vi "Grid_multiGrid_v8.vi"() -> ()   [LabVIEW 2014]
uses:
  <userlib>/Nanonis Prog Interface V5/Nanonis Prog Interface.lvlib
panel:
  out "size(s) 5":i32
  out "size(s) 4":i32
  out "size(s) 3":i32=11
  out "size(s) 2":i32=12
  out "size(s)":i32=15
  out "data\n\n 5":T1(array[cluster])=[{"Amplitude (mod. signal unit)"=0.0, "Lockin on/off status"=FALSE, "Backward sweep"=TRUE, "Number of points"=215, "Channels"=["Current (A)", "LI Demod 1 X (A)", "LI Demod 1 Y (A)", "LI Demod 2 X (A)", "LI Demod 2 Y (A)"], "Parameters"=["X (m)", "Y (m)", "Z (m)", "Z offset (m)", "Settling time (s)", "Integration time (s)", "Z-Ctrl hold", "Final Z (m)"], "Fixed parameters"=["Sweep Start", "Sweep End"], "Multiple sweeps configuration"={"Number of Sweeps"=1, "Save all"=FALSE}, "Initialization"={"Z averaging time (s)"=0.001, "Initial settling time (s)"=0.0002}, "Sweep Timing"={"Max. slew rate (V/s)"=inf, "Settling time (s)"=0.001, "Integration time (s)"=0.001}, "End of Sweep"={"End settling time (s)"=5e-05, "Z control time (s)"=0.0002}, "Initial Z-Offset (m)"=0.0, "Sweep Distance (m)"=0.0, "Channels 2"=[], "Name"="", "Reset Z"=FALSE, "Record final Z"=FALSE, "Auto Retract Status"=FALSE, "Threshold"=0.0, "Auto Retract Signal Index"=0, "Auto Retract Condition"=FALSE}, {"Amplitude (mod. signal unit)"=0.0, "Lockin on/off status"=FALSE, "Backward sweep"=FALSE, "Number of points"=0, "Channels"=[], "Parameters"=[], "Fixed parameters"=[], "Multiple sweeps configuration"={"Number of Sweeps"=0, "Save all"=FALSE}, "Initialization"={"Z averaging time (s)"=0.0, "Initial settling time (s)"=0.0}, "Sweep Timing"={"Max. slew rate (V/s)"=0.0, "Settling time (s)"=0.0, "Integration time (s)"=0.0}, "End of Sweep"={"End settling time (s)"=0.0, "Z control time (s)"=0.0}, "Initial Z-Offset (m)"=0.0, "Sweep Distance (m)"=0.0, "Channels 2"=[], "Name"="", "Reset Z"=FALSE, "Record final Z"=FALSE, "Auto Retract Status"=FALSE, "Threshold"=0.0, "Auto Retract Signal Index"=0, "Auto Retract Condition"=FALSE}, {"Amplitude (mod. signal unit)"=0.0, "Lockin on/off status"=FALSE, "Backward sweep"=FALSE, "Number of points"=0, "Channels"=[], "Parameters"=[], "Fixed parameters"=[], "Multiple sweeps configuration"={"Number of Sweeps"=0, "Save all"=FALSE}, "Initialization"={"Z averaging time (s)"=0.0, "Initial settling time (s)"=0.0}, "Sweep Timing"={"Max. slew rate (V/s)"=0.0, "Settling time (s)"=0.0, "Integration time (s)"=0.0}, "End of Sweep"={"End settling time (s)"=0.0, "Z control time (s)"=0.0}, "Initial Z-Offset (m)"=0.0, "Sweep Distance (m)"=0.0, "Channels 2"=[], "Name"="", "Reset Z"=FALSE, "Record final Z"=FALSE, "Auto Retract Status"=FALSE, "Threshold"=0.0, "Auto Retract Signal Index"=0, "Auto Retract Condition"=FALSE}, {"Amplitude (mod. signal unit)"=0.0, "Lockin on/off status"=FALSE, "Backward sweep"=FALSE, "Number of points"=0, "Channels"=[], "Parameters"=[], "Fixed parameters"=[], "Multiple sweeps configuration"={"Number of Sweeps"=0, "Save all"=FALSE}, "Initialization"={"Z averaging time (s)"=0.0, "Initial settling time (s)"=0.0}, "Sweep Timing"={"Max. slew rate (V/s)"=0.0, "Settling time (s)"=0.0, "Integration time (s)"=0.0}, "End of Sweep"={"End settling time (s)"=0.0, "Z control time (s)"=0.0}, "Initial Z-Offset (m)"=0.0, "Sweep Distance (m)"=0.0, "Channels 2"=[], "Name"="", "Reset Z"=FALSE, "Record final Z"=FALSE, "Auto Retract Status"=FALSE, "Threshold"=0.0, "Auto Retract Signal Index"=0, "Auto Retract Condition"=FALSE}, {"Amplitude (mod. signal unit)"=0.0, "Lockin on/off status"=FALSE, "Backward sweep"=FALSE, "Number of points"=0, "Channels"=[], "Parameters"=[], "Fixed parameters"=[], "Multiple sweeps configuration"={"Number of Sweeps"=0, "Save all"=FALSE}, "Initialization"={"Z averaging time (s)"=0.0, "Initial settling time (s)"=0.0}, "Sweep Timing"={"Max. slew rate (V/s)"=0.0, "Settling time (s)"=0.0, "Integration time (s)"=0.0}, "End of Sweep"={"End settling time (s)"=0.0, "Z control time (s)"=0.0}, "Initial Z-Offset (m)"=0.0, "Sweep Distance (m)"=0.0, "Channels 2"=[], "Name"="", "Reset Z"=FALSE, "Record final Z"=FALSE, "Auto Retract Status"=FALSE, "Threshold"=0.0, "Auto Retract Signal Index"=0, "Auto Retract Condition"=FALSE}, {"Amplitude (mod. signal unit)"=0.0, "Lockin on/off status"=FALSE, "Backward sweep"=FALSE, "Number of points"=0, "Channels"=[], "Parameters"=[], "Fixed parameters"=[], "Multiple sweeps configuration"={"Number of Sweeps"=0, "Save all"=FALSE}, "Initialization"={"Z averaging time (s)"=0.0, "Initial settling time (s)"=0.0}, "Sweep Timing"={"Max. slew rate (V/s)"=0.0, "Settling time (s)"=0.0, "Integration time (s)"=0.0}, "End of Sweep"={"End settling time (s)"=0.0, "Z control time (s)"=0.0}, "Initial Z-Offset (m)"=0.0, "Sweep Distance (m)"=0.0, "Channels 2"=[], "Name"="", "Reset Z"=FALSE, "Record final Z"=FALSE, "Auto Retract Status"=FALSE, "Threshold"=0.0, "Auto Retract Signal Index"=0, "Auto Retract Condition"=FALSE}, {"Amplitude (mod. signal unit)"=0.0, "Lockin on/off status"=FALSE, "Backward sweep"=FALSE, "Number of points"=0, "Channels"=[], "Parameters"=[], "Fixed parameters"=[], "Multiple sweeps configuration"={"Number of Sweeps"=0, "Save all"=FALSE}, "Initialization"={"Z averaging time (s)"=0.0, "Initial settling time (s)"=0.0}, "Sweep Timing"={"Max. slew rate (V/s)"=0.0, "Settling time (s)"=0.0, "Integration time (s)"=0.0}, "End of Sweep"={"End settling time (s)"=0.0, "Z control time (s)"=0.0}, "Initial Z-Offset (m)"=0.0, "Sweep Distance (m)"=0.0, "Channels 2"=[], "Name"="", "Reset Z"=FALSE, "Record final Z"=FALSE, "Auto Retract Status"=FALSE, "Threshold"=0.0, "Auto Retract Signal Index"=0, "Auto Retract Condition"=FALSE}, {"Amplitude (mod. signal unit)"=0.0, "Lockin on/off status"=FALSE, "Backward sweep"=FALSE, "Number of points"=0, "Channels"=[], "Parameters"=[], "Fixed parameters"=[], "Multiple sweeps configuration"={"Number of Sweeps"=0, "Save all"=FALSE}, "Initialization"={"Z averaging time (s)"=0.0, "Initial settling time (s)"=0.0}, "Sweep Timing"={"Max. slew rate (V/s)"=0.0, "Settling time (s)"=0.0, "Integration time (s)"=0.0}, "End of Sweep"={"End settling time (s)"=0.0, "Z control time (s)"=0.0}, "Initial Z-Offset (m)"=0.0, "Sweep Distance (m)"=0.0, "Channels 2"=[], "Name"="", "Reset Z"=FALSE, "Record final Z"=FALSE, "Auto Retract Status"=FALSE, "Threshold"=0.0, "Auto Retract Signal Index"=0, "Auto Retract Condition"=FALSE}, {"Amplitude (mod. signal unit)"=0.0, "Lockin on/off status"=FALSE, "Backward sweep"=FALSE, "Number of points"=0, "Channels"=[], "Parameters"=[], "Fixed parameters"=[], "Multiple sweeps configuration"={"Number of Sweeps"=0, "Save all"=FALSE}, "Initialization"={"Z averaging time (s)"=0.0, "Initial settling time (s)"=0.0}, "Sweep Timing"={"Max. slew rate (V/s)"=0.0, "Settling time (s)"=0.0, "Integration time (s)"=0.0}, "End of Sweep"={"End settling time (s)"=0.0, "Z control time (s)"=0.0}, "Initial Z-Offset (m)"=0.0, "Sweep Distance (m)"=0.0, "Channels 2"=[], "Name"="", "Reset Z"=FALSE, "Record final Z"=FALSE, "Auto Retract Status"=FALSE, "Threshold"=0.0, "Auto Retract Signal Index"=0, "Auto Retract Condition"=FALSE}, {"Amplitude (mod. signal unit)"=0.0, "Lockin on/off status"=FALSE, "Backward sweep"=FALSE, "Number of points"=0, "Channels"=[], "Parameters"=[], "Fixed parameters"=[], "Multiple sweeps configuration"={"Number of Sweeps"=0, "Save all"=FALSE}, "Initialization"={"Z averaging time (s)"=0.0, "Initial settling time (s)"=0.0}, "Sweep Timing"={"Max. slew rate (V/s)"=0.0, "Settling time (s)"=0.0, "Integration time (s)"=0.0}, "End of Sweep"={"End settling time (s)"=0.0, "Z control time (s)"=0.0}, "Initial Z-Offset (m)"=0.0, "Sweep Distance (m)"=0.0, "Channels 2"=[], "Name"="", "Reset Z"=FALSE, "Record final Z"=FALSE, "Auto Retract Status"=FALSE, "Threshold"=0.0, "Auto Retract Signal Index"=0, "Auto Retract Condition"=FALSE}, {"Amplitude (mod. signal unit)"=0.0, "Lockin on/off status"=FALSE, "Backward sweep"=FALSE, "Number of points"=0, "Channels"=[], "Parameters"=[], "Fixed parameters"=[], "Multiple sweeps configuration"={"Number of Sweeps"=0, "Save all"=FALSE}, "Initialization"={"Z averaging time (s)"=0.0, "Initial settling time (s)"=0.0}, "Sweep Timing"={"Max. slew rate (V/s)"=0.0, "Settling time (s)"=0.0, "Integration time (s)"=0.0}, "End of Sweep"={"End settling time (s)"=0.0, "Z control time (s)"=0.0}, "Initial Z-Offset (m)"=0.0, "Sweep Distance (m)"=0.0, "Channels 2"=[], "Name"="", "Reset Z"=FALSE, "Record final Z"=FALSE, "Auto Retract Status"=FALSE, "Threshold"=0.0, "Auto Retract Signal Index"=0, "Auto Retract Condition"=FALSE}, {"Amplitude (mod. signal unit)"=0.0, "Lockin on/off status"=FALSE, "Backward sweep"=FALSE, "Number of points"=0, "Channels"=[], "Parameters"=[], "Fixed parameters"=[], "Multiple sweeps configuration"={"Number of Sweeps"=0, "Save all"=FALSE}, "Initialization"={"Z averaging time (s)"=0.0, "Initial settling time (s)"=0.0}, "Sweep Timing"={"Max. slew rate (V/s)"=0.0, "Settling time (s)"=0.0, "Integration time (s)"=0.0}, "End of Sweep"={"End settling time (s)"=0.0, "Z control time (s)"=0.0}, "Initial Z-Offset (m)"=0.0, "Sweep Distance (m)"=0.0, "Channels 2"=[], "Name"="", "Reset Z"=FALSE, "Record final Z"=FALSE, "Auto Retract Status"=FALSE, "Threshold"=0.0, "Auto Retract Signal Index"=0, "Auto Retract Condition"=FALSE}, {"Amplitude (mod. signal unit)"=0.0, "Lockin on/off status"=FALSE, "Backward sweep"=FALSE, "Number of points"=0, "Channels"=[], "Parameters"=[], "Fixed parameters"=[], "Multiple sweeps configuration"={"Number of Sweeps"=0, "Save all"=FALSE}, "Initialization"={"Z averaging time (s)"=0.0, "Initial settling time (s)"=0.0}, "Sweep Timing"={"Max. slew rate (V/s)"=0.0, "Settling time (s)"=0.0, "Integration time (s)"=0.0}, "End of Sweep"={"End settling time (s)"=0.0, "Z control time (s)"=0.0}, "Initial Z-Offset (m)"=0.0, "Sweep Distance (m)"=0.0, "Channels 2"=[], "Name"="", "Reset Z"=FALSE, "Record final Z"=FALSE, "Auto Retract Status"=FALSE, "Threshold"=0.0, "Auto Retract Signal Index"=0, "Auto Retract Condition"=FALSE}, {"Amplitude (mod. signal unit)"=0.0, "Lockin on/off status"=FALSE, "Backward sweep"=FALSE, "Number of points"=0, "Channels"=[], "Parameters"=[], "Fixed parameters"=[], "Multiple sweeps configuration"={"Number of Sweeps"=0, "Save all"=FALSE}, "Initialization"={"Z averaging time (s)"=0.0, "Initial settling time (s)"=0.0}, "Sweep Timing"={"Max. slew rate (V/s)"=0.0, "Settling time (s)"=0.0, "Integration time (s)"=0.0}, "End of Sweep"={"End settling time (s)"=0.0, "Z control time (s)"=0.0}, "Initial Z-Offset (m)"=0.0, "Sweep Distance (m)"=0.0, "Channels 2"=[], "Name"="", "Reset Z"=FALSE, "Record final Z"=FALSE, "Auto Retract Status"=FALSE, "Threshold"=0.0, "Auto Retract Signal Index"=0, "Auto Retract Condition"=FALSE}, {"Amplitude (mod. signal unit)"=0.0, "Lockin on/off status"=FALSE, "Backward sweep"=FALSE, "Number of points"=0, "Channels"=[], "Parameters"=[], "Fixed parameters"=[], "Multiple sweeps configuration"={"Number of Sweeps"=0, "Save all"=FALSE}, "Initialization"={"Z averaging time (s)"=0.0, "Initial settling time (s)"=0.0}, "Sweep Timing"={"Max. slew rate (V/s)"=0.0, "Settling time (s)"=0.0, "Integration time (s)"=0.0}, "End of Sweep"={"End settling time (s)"=0.0, "Z control time (s)"=0.0}, "Initial Z-Offset (m)"=0.0, "Sweep Distance (m)"=0.0, "Channels 2"=[], "Name"="", "Reset Z"=FALSE, "Record final Z"=FALSE, "Auto Retract Status"=FALSE, "Threshold"=0.0, "Auto Retract Signal Index"=0, "Auto Retract Condition"=FALSE}, {"Amplitude (mod. signal unit)"=0.0, "Lockin on/off status"=FALSE, "Backward sweep"=FALSE, "Number of points"=0, "Channels"=[], "Parameters"=[], "Fixed parameters"=[], "Multiple sweeps configuration"={"Number of Sweeps"=0, "Save all"=FALSE}, "Initialization"={"Z averaging time (s)"=0.0, "Initial settling time (s)"=0.0}, "Sweep Timing"={"Max. slew rate (V/s)"=0.0, "Settling time (s)"=0.0, "Integration time (s)"=0.0}, "End of Sweep"={"End settling time (s)"=0.0, "Z control time (s)"=0.0}, "Initial Z-Offset (m)"=0.0, "Sweep Distance (m)"=0.0, "Channels 2"=[], "Name"="", "Reset Z"=FALSE, "Record final Z"=FALSE, "Auto Retract Status"=FALSE, "Threshold"=0.0, "Auto Retract Signal Index"=0, "Auto Retract Condition"=FALSE}, {"Amplitude (mod. signal unit)"=0.0, "Lockin on/off status"=FALSE, "Backward sweep"=FALSE, "Number of points"=0, "Channels"=[], "Parameters"=[], "Fixed parameters"=[], "Multiple sweeps configuration"={"Number of Sweeps"=0, "Save all"=FALSE}, "Initialization"={"Z averaging time (s)"=0.0, "Initial settling time (s)"=0.0}, "Sweep Timing"={"Max. slew rate (V/s)"=0.0, "Settling time (s)"=0.0, "Integration time (s)"=0.0}, "End of Sweep"={"End settling time (s)"=0.0, "Z control time (s)"=0.0}, "Initial Z-Offset (m)"=0.0, "Sweep Distance (m)"=0.0, "Channels 2"=[], "Name"="", "Reset Z"=FALSE, "Record final Z"=FALSE, "Auto Retract Status"=FALSE, "Threshold"=0.0, "Auto Retract Signal Index"=0, "Auto Retract Condition"=FALSE}, {"Amplitude (mod. signal unit)"=0.0, "Lockin on/off status"=FALSE, "Backward sweep"=FALSE, "Number of points"=0, "Channels"=[], "Parameters"=[], "Fixed parameters"=[], "Multiple sweeps configuration"={"Number of Sweeps"=0, "Save all"=FALSE}, "Initialization"={"Z averaging time (s)"=0.0, "Initial settling time (s)"=0.0}, "Sweep Timing"={"Max. slew rate (V/s)"=0.0, "Settling time (s)"=0.0, "Integration time (s)"=0.0}, "End of Sweep"={"End settling time (s)"=0.0, "Z control time (s)"=0.0}, "Initial Z-Offset (m)"=0.0, "Sweep Distance (m)"=0.0, "Channels 2"=[], "Name"="", "Reset Z"=FALSE, "Record final Z"=FALSE, "Auto Retract Status"=FALSE, "Threshold"=0.0, "Auto Retract Signal Index"=0, "Auto Retract Condition"=FALSE}]
  out "data\n\n 2":T2(array[cluster])=[{"Amplitude (mod. signal unit)"=0.0, "Lockin on/off status"=FALSE, "Advanced options"={"Z-Controller Hold"=TRUE, "Record final Z"=FALSE, "Reset Bias"=TRUE}, "Backward sweep"=TRUE, "Number of points"=215, "Channels"=["Current (A)", "LI Demod 1 X (A)", "LI Demod 1 Y (A)", "LI Demod 2 X (A)", "LI Demod 2 Y (A)"], "Parameters"=["X (m)", "Y (m)", "Z (m)", "Z offset (m)", "Settling time (s)", "Integration time (s)", "Z-Ctrl hold", "Final Z (m)"], "Fixed parameters"=["Sweep Start", "Sweep End"], "Multiple sweeps configuration"={"Number of Sweeps"=1, "Save all"=FALSE}, "Initialization"={"Z averaging time (s)"=0.001, "Z offset (m)"=0.0, "Initial settling time (s)"=0.0002}, "Sweep Timing"={"Max. slew rate (V/s)"=inf, "Settling time (s)"=0.001, "Integration time (s)"=0.001}, "End of Sweep"={"End settling time (s)"=5e-05, "Z control time (s)"=0.0002}, "Start value (V)"=-0.02, "End value (V)"=-3.0, "Channels 2"=[0, 20, 21, 22, 23], "Name"="numerical_DCA_-20mV->-3V"}, {"Amplitude (mod. signal unit)"=0.0, "Lockin on/off status"=FALSE, "Advanced options"={"Z-Controller Hold"=TRUE, "Record final Z"=FALSE, "Reset Bias"=TRUE}, "Backward sweep"=TRUE, "Number of points"=215, "Channels"=["Current (A)", "LI Demod 1 X (A)", "LI Demod 1 Y (A)", "LI Demod 2 X (A)", "LI Demod 2 Y (A)"], "Parameters"=["X (m)", "Y (m)", "Z (m)", "Z offset (m)", "Settling time (s)", "Integration time (s)", "Z-Ctrl hold", "Final Z (m)"], "Fixed parameters"=["Sweep Start", "Sweep End"], "Multiple sweeps configuration"={"Number of Sweeps"=1, "Save all"=FALSE}, "Initialization"={"Z averaging time (s)"=0.001, "Z offset (m)"=0.0, "Initial settling time (s)"=0.0002}, "Sweep Timing"={"Max. slew rate (V/s)"=inf, "Settling time (s)"=0.001, "Integration time (s)"=0.001}, "End of Sweep"={"End settling time (s)"=5e-05, "Z control time (s)"=0.0002}, "Start value (V)"=-0.02, "End value (V)"=0.7, "Channels 2"=[0, 20, 21, 22, 23], "Name"="numerical_DCA_-20mV->0.7V"}, {"Amplitude (mod. signal unit)"=0.0, "Lockin on/off status"=FALSE, "Advanced options"={"Z-Controller Hold"=TRUE, "Record final Z"=FALSE, "Reset Bias"=TRUE}, "Backward sweep"=TRUE, "Number of points"=215, "Channels"=["Current (A)", "LI Demod 1 X (A)", "LI Demod 1 Y (A)", "LI Demod 2 X (A)", "LI Demod 2 Y (A)"], "Parameters"=["X (m)", "Y (m)", "Z (m)", "Z offset (m)", "Settling time (s)", "Integration time (s)", "Z-Ctrl hold", "Final Z (m)"], "Fixed parameters"=["Sweep Start", "Sweep End"], "Multiple sweeps configuration"={"Number of Sweeps"=30, "Save all"=FALSE}, "Initialization"={"Z averaging time (s)"=0.001, "Z offset (m)"=0.0, "Initial settling time (s)"=0.0002}, "Sweep Timing"={"Max. slew rate (V/s)"=inf, "Settling time (s)"=0.001, "Integration time (s)"=0.001}, "End of Sweep"={"End settling time (s)"=5e-05, "Z control time (s)"=0.0002}, "Start value (V)"=-0.02, "End value (V)"=0.7, "Channels 2"=[0, 20, 21, 22, 23], "Name"="numerical_DCA_-20mV->-0.7V_30sweeps"}, {"Amplitude (mod. signal unit)"=0.0, "Lockin on/off status"=FALSE, "Advanced options"={"Z-Controller Hold"=TRUE, "Record final Z"=FALSE, "Reset Bias"=TRUE}, "Backward sweep"=TRUE, "Number of points"=215, "Channels"=["Current (A)", "LI Demod 1 X (A)", "LI Demod 1 Y (A)", "LI Demod 2 X (A)", "LI Demod 2 Y (A)"], "Parameters"=["X (m)", "Y (m)", "Z (m)", "Z offset (m)", "Settling time (s)", "Integration time (s)", "Z-Ctrl hold", "Final Z (m)"], "Fixed parameters"=["Sweep Start", "Sweep End"], "Multiple sweeps configuration"={"Number of Sweeps"=50, "Save all"=FALSE}, "Initialization"={"Z averaging time (s)"=0.001, "Z offset (m)"=0.0, "Initial settling time (s)"=0.0002}, "Sweep Timing"={"Max. slew rate (V/s)"=inf, "Settling time (s)"=0.001, "Integration time (s)"=0.001}, "End of Sweep"={"End settling time (s)"=5e-05, "Z control time (s)"=0.0002}, "Start value (V)"=-0.02, "End value (V)"=0.7, "Channels 2"=[0, 20, 21, 22, 23], "Name"="numerical_DCA_-20mV->-0.7V_50_sweeps"}, {"Amplitude (mod. signal unit)"=0.0, "Lockin on/off status"=FALSE, "Advanced options"={"Z-Controller Hold"=TRUE, "Record final Z"=FALSE, "Reset Bias"=TRUE}, "Backward sweep"=TRUE, "Number of points"=215, "Channels"=["Current (A)", "LI Demod 1 X (A)", "LI Demod 1 Y (A)", "LI Demod 2 X (A)", "LI Demod 2 Y (A)"], "Parameters"=["X (m)", "Y (m)", "Z (m)", "Z offset (m)", "Settling time (s)", "Integration time (s)", "Z-Ctrl hold", "Final Z (m)"], "Fixed parameters"=["Sweep Start", "Sweep End"], "Multiple sweeps configuration"={"Number of Sweeps"=70, "Save all"=FALSE}, "Initialization"={"Z averaging time (s)"=0.001, "Z offset (m)"=0.0, "Initial settling time (s)"=0.0002}, "Sweep Timing"={"Max. slew rate (V/s)"=inf, "Settling time (s)"=0.001, "Integration time (s)"=0.001}, "End of Sweep"={"End settling time (s)"=5e-05, "Z control time (s)"=0.0002}, "Start value (V)"=-0.02, "End value (V)"=-3.0, "Channels 2"=[0, 20, 21, 22, 23], "Name"="numerical_DCA_-20mV->-3V_70sweeps"}, {"Amplitude (mod. signal unit)"=0.0, "Lockin on/off status"=FALSE, "Advanced options"={"Z-Controller Hold"=TRUE, "Record final Z"=FALSE, "Reset Bias"=TRUE}, "Backward sweep"=TRUE, "Number of points"=215, "Channels"=["Current (A)", "LI Demod 1 X (A)", "LI Demod 1 Y (A)", "LI Demod 2 X (A)", "LI Demod 2 Y (A)"], "Parameters"=["X (m)", "Y (m)", "Z (m)", "Z offset (m)", "Settling time (s)", "Integration time (s)", "Z-Ctrl hold", "Final Z (m)"], "Fixed parameters"=["Sweep Start", "Sweep End"], "Multiple sweeps configuration"={"Number of Sweeps"=100, "Save all"=FALSE}, "Initialization"={"Z averaging time (s)"=0.001, "Z offset (m)"=0.0, "Initial settling time (s)"=0.0002}, "Sweep Timing"={"Max. slew rate (V/s)"=inf, "Settling time (s)"=0.001, "Integration time (s)"=0.001}, "End of Sweep"={"End settling time (s)"=5e-05, "Z control time (s)"=0.0002}, "Start value (V)"=-0.02, "End value (V)"=-3.0, "Channels 2"=[0, 20, 21, 22, 23], "Name"="numerical_DCA_-20mV->3V_100_sweeps"}, {"Amplitude (mod. signal unit)"=0.0, "Lockin on/off status"=FALSE, "Advanced options"={"Z-Controller Hold"=TRUE, "Record final Z"=FALSE, "Reset Bias"=TRUE}, "Backward sweep"=TRUE, "Number of points"=256, "Channels"=["Current (A)", "LI Demod 1 X (A)", "LI Demod 1 Y (A)", "LI Demod 2 X (A)", "LI Demod 2 Y (A)"], "Parameters"=["X (m)", "Y (m)", "Z (m)", "Z offset (m)", "Settling time (s)", "Integration time (s)", "Z-Ctrl hold", "Final Z (m)"], "Fixed parameters"=["Sweep Start", "Sweep End"], "Multiple sweeps configuration"={"Number of Sweeps"=100, "Save all"=FALSE}, "Initialization"={"Z averaging time (s)"=0.001, "Z offset (m)"=0.0, "Initial settling time (s)"=5e-05}, "Sweep Timing"={"Max. slew rate (V/s)"=inf, "Settling time (s)"=0.001, "Integration time (s)"=0.0005}, "End of Sweep"={"End settling time (s)"=5e-05, "Z control time (s)"=5e-05}, "Start value (V)"=-1.0, "End value (V)"=2.0, "Channels 2"=[0, 20, 21, 22, 23], "Name"="numerical_-1V->2V"}, {"Amplitude (mod. signal unit)"=0.0, "Lockin on/off status"=FALSE, "Advanced options"={"Z-Controller Hold"=TRUE, "Record final Z"=FALSE, "Reset Bias"=TRUE}, "Backward sweep"=TRUE, "Number of points"=256, "Channels"=["Current (A)", "LI Demod 1 X (A)", "LI Demod 1 Y (A)", "LI Demod 2 X (A)", "LI Demod 2 Y (A)"], "Parameters"=["X (m)", "Y (m)", "Z (m)", "Z offset (m)", "Settling time (s)", "Integration time (s)", "Z-Ctrl hold", "Final Z (m)"], "Fixed parameters"=["Sweep Start", "Sweep End"], "Multiple sweeps configuration"={"Number of Sweeps"=100, "Save all"=FALSE}, "Initialization"={"Z averaging time (s)"=0.001, "Z offset (m)"=0.0, "Initial settling time (s)"=5e-05}, "Sweep Timing"={"Max. slew rate (V/s)"=inf, "Settling time (s)"=0.001, "Integration time (s)"=0.0005}, "End of Sweep"={"End settling time (s)"=5e-05, "Z control time (s)"=5e-05}, "Start value (V)"=-0.02, "End value (V)"=0.02, "Channels 2"=[0, 20, 21, 22, 23], "Name"="numerical_-20mV->20mV"}, {"Amplitude (mod. signal unit)"=0.0, "Lockin on/off status"=FALSE, "Advanced options"={"Z-Controller Hold"=TRUE, "Record final Z"=FALSE, "Reset Bias"=TRUE}, "Backward sweep"=TRUE, "Number of points"=286, "Channels"=["Current (A)", "LI Demod 1 X (A)", "LI Demod 1 Y (A)", "LI Demod 2 X (A)", "LI Demod 2 Y (A)"], "Parameters"=["X (m)", "Y (m)", "Z (m)", "Z offset (m)", "Settling time (s)", "Integration time (s)", "Z-Ctrl hold", "Final Z (m)"], "Fixed parameters"=["Sweep Start", "Sweep End"], "Multiple sweeps configuration"={"Number of Sweeps"=50, "Save all"=FALSE}, "Initialization"={"Z averaging time (s)"=0.001, "Z offset (m)"=0.0, "Initial settling time (s)"=5e-05}, "Sweep Timing"={"Max. slew rate (V/s)"=inf, "Settling time (s)"=0.001, "Integration time (s)"=0.0005}, "End of Sweep"={"End settling time (s)"=5e-05, "Z control time (s)"=5e-05}, "Start value (V)"=-0.2, "End value (V)"=0.8, "Channels 2"=[0, 20, 21, 22, 23], "Name"="DCA_numerical_-0.2V->0.8V"}, {"Amplitude (mod. signal unit)"=0.0, "Lockin on/off status"=FALSE, "Advanced options"={"Z-Controller Hold"=TRUE, "Record final Z"=FALSE, "Reset Bias"=TRUE}, "Backward sweep"=TRUE, "Number of points"=421, "Channels"=["Current (A)", "LI Demod 1 X (A)", "LI Demod 1 Y (A)", "LI Demod 2 X (A)", "LI Demod 2 Y (A)"], "Parameters"=["X (m)", "Y (m)", "Z (m)", "Z offset (m)", "Settling time (s)", "Integration time (s)", "Z-Ctrl hold", "Final Z (m)"], "Fixed parameters"=["Sweep Start", "Sweep End"], "Multiple sweeps configuration"={"Number of Sweeps"=100, "Save all"=FALSE}, "Initialization"={"Z averaging time (s)"=0.001, "Z offset (m)"=0.0, "Initial settling time (s)"=5e-05}, "Sweep Timing"={"Max. slew rate (V/s)"=inf, "Settling time (s)"=0.001, "Integration time (s)"=0.0005}, "End of Sweep"={"End settling time (s)"=5e-05, "Z control time (s)"=5e-05}, "Start value (V)"=-2.0, "End value (V)"=2.2, "Channels 2"=[0, 20, 21, 22, 23], "Name"="numerical_-2V->2.2V"}, {"Amplitude (mod. signal unit)"=0.0, "Lockin on/off status"=FALSE, "Advanced options"={"Z-Controller Hold"=TRUE, "Record final Z"=FALSE, "Reset Bias"=TRUE}, "Backward sweep"=TRUE, "Number of points"=500, "Channels"=["Current (A)", "LI Demod 1 X (A)", "LI Demod 1 Y (A)", "LI Demod 2 X (A)", "LI Demod 2 Y (A)"], "Parameters"=["X (m)", "Y (m)", "Z (m)", "Z offset (m)", "Settling time (s)", "Integration time (s)", "Z-Ctrl hold", "Final Z (m)"], "Fixed parameters"=["Sweep Start", "Sweep End"], "Multiple sweeps configuration"={"Number of Sweeps"=20, "Save all"=FALSE}, "Initialization"={"Z averaging time (s)"=0.001, "Z offset (m)"=0.0, "Initial settling time (s)"=0.01}, "Sweep Timing"={"Max. slew rate (V/s)"=inf, "Settling time (s)"=0.001, "Integration time (s)"=0.001}, "End of Sweep"={"End settling time (s)"=0.1, "Z control time (s)"=0.001}, "Start value (V)"=-0.2, "End value (V)"=0.8, "Channels 2"=[0, 20, 21, 22, 23], "Name"="DCA_numerical2_-0.2V->0.8V"}, {"Amplitude (mod. signal unit)"=0.0015, "Lockin on/off status"=FALSE, "Advanced options"={"Z-Controller Hold"=TRUE, "Record final Z"=FALSE, "Reset Bias"=TRUE}, "Backward sweep"=TRUE, "Number of points"=80, "Channels"=["Current (A)", "LI Demod 1 X (A)", "LI Demod 1 Y (A)", "LI Demod 2 X (A)", "LI Demod 2 Y (A)"], "Parameters"=["X (m)", "Y (m)", "Z (m)", "Z offset (m)", "Settling time (s)", "Integration time (s)", "Z-Ctrl hold", "Final Z (m)"], "Fixed parameters"=["Sweep Start", "Sweep End"], "Multiple sweeps configuration"={"Number of Sweeps"=10, "Save all"=FALSE}, "Initialization"={"Z averaging time (s)"=0.001, "Z offset (m)"=0.0, "Initial settling time (s)"=0.0046}, "Sweep Timing"={"Max. slew rate (V/s)"=inf, "Settling time (s)"=0.0046, "Integration time (s)"=0.032}, "End of Sweep"={"End settling time (s)"=5e-05, "Z control time (s)"=5e-05}, "Start value (V)"=-0.02, "End value (V)"=0.02, "Channels 2"=[0, 20, 21, 22, 23], "Name"="lockin_-20mV->20mV"}, {"Amplitude (mod. signal unit)"=0.002, "Lockin on/off status"=FALSE, "Advanced options"={"Z-Controller Hold"=TRUE, "Record final Z"=FALSE, "Reset Bias"=TRUE}, "Backward sweep"=TRUE, "Number of points"=70, "Channels"=["Current (A)", "LI Demod 1 X (A)", "LI Demod 1 Y (A)", "LI Demod 2 X (A)", "LI Demod 2 Y (A)"], "Parameters"=["X (m)", "Y (m)", "Z (m)", "Z offset (m)", "Settling time (s)", "Integration time (s)", "Z-Ctrl hold", "Final Z (m)"], "Fixed parameters"=["Sweep Start", "Sweep End"], "Multiple sweeps configuration"={"Number of Sweeps"=10, "Save all"=FALSE}, "Initialization"={"Z averaging time (s)"=0.001, "Z offset (m)"=0.0, "Initial settling time (s)"=0.0046}, "Sweep Timing"={"Max. slew rate (V/s)"=inf, "Settling time (s)"=0.0046, "Integration time (s)"=0.032}, "End of Sweep"={"End settling time (s)"=5e-05, "Z control time (s)"=5e-05}, "Start value (V)"=-0.025, "End value (V)"=0.025, "Channels 2"=[0, 20, 21, 22, 23], "Name"="lockin_-25mV->25mV"}, {"Amplitude (mod. signal unit)"=0.002, "Lockin on/off status"=FALSE, "Advanced options"={"Z-Controller Hold"=TRUE, "Record final Z"=FALSE, "Reset Bias"=TRUE}, "Backward sweep"=TRUE, "Number of points"=70, "Channels"=["Current (A)", "LI Demod 1 X (A)", "LI Demod 1 Y (A)", "LI Demod 2 X (A)", "LI Demod 2 Y (A)"], "Parameters"=["X (m)", "Y (m)", "Z (m)", "Z offset (m)", "Settling time (s)", "Integration time (s)", "Z-Ctrl hold", "Final Z (m)"], "Fixed parameters"=["Sweep Start", "Sweep End"], "Multiple sweeps configuration"={"Number of Sweeps"=10, "Save all"=FALSE}, "Initialization"={"Z averaging time (s)"=0.001, "Z offset (m)"=0.0, "Initial settling time (s)"=0.0046}, "Sweep Timing"={"Max. slew rate (V/s)"=inf, "Settling time (s)"=0.0046, "Integration time (s)"=0.032}, "End of Sweep"={"End settling time (s)"=5e-05, "Z control time (s)"=5e-05}, "Start value (V)"=-0.025, "End value (V)"=0.025, "Channels 2"=[0, 20, 21, 22, 23], "Name"="test"}, {"Amplitude (mod. signal unit)"=0.0025, "Lockin on/off status"=FALSE, "Advanced options"={"Z-Controller Hold"=TRUE, "Record final Z"=FALSE, "Reset Bias"=TRUE}, "Backward sweep"=TRUE, "Number of points"=320, "Channels"=["Current (A)", "LI Demod 1 X (A)", "LI Demod 1 Y (A)", "LI Demod 2 X (A)", "LI Demod 2 Y (A)"], "Parameters"=["X (m)", "Y (m)", "Z (m)", "Z offset (m)", "Settling time (s)", "Integration time (s)", "Z-Ctrl hold", "Final Z (m)"], "Fixed parameters"=["Sweep Start", "Sweep End"], "Multiple sweeps configuration"={"Number of Sweeps"=1, "Save all"=FALSE}, "Initialization"={"Z averaging time (s)"=0.001, "Z offset (m)"=0.0, "Initial settling time (s)"=0.0046}, "Sweep Timing"={"Max. slew rate (V/s)"=inf, "Settling time (s)"=0.0046, "Integration time (s)"=0.0042}, "End of Sweep"={"End settling time (s)"=5e-05, "Z control time (s)"=5e-05}, "Start value (V)"=0.02, "End value (V)"=-0.02, "Channels 2"=[0, 20, 21, 22, 23], "Name"="lockin_highRes_20mV_-20mV"}, {"Amplitude (mod. signal unit)"=0.005, "Lockin on/off status"=FALSE, "Advanced options"={"Z-Controller Hold"=TRUE, "Record final Z"=FALSE, "Reset Bias"=TRUE}, "Backward sweep"=TRUE, "Number of points"=256, "Channels"=["Current (A)", "LI Demod 1 X (A)", "LI Demod 1 Y (A)", "LI Demod 2 X (A)", "LI Demod 2 Y (A)"], "Parameters"=["X (m)", "Y (m)", "Z (m)", "Z offset (m)", "Settling time (s)", "Integration time (s)", "Z-Ctrl hold", "Final Z (m)"], "Fixed parameters"=["Sweep Start", "Sweep End"], "Multiple sweeps configuration"={"Number of Sweeps"=2, "Save all"=FALSE}, "Initialization"={"Z averaging time (s)"=0.001, "Z offset (m)"=0.0, "Initial settling time (s)"=0.0033}, "Sweep Timing"={"Max. slew rate (V/s)"=inf, "Settling time (s)"=0.0033, "Integration time (s)"=0.0164}, "End of Sweep"={"End settling time (s)"=5e-05, "Z control time (s)"=5e-05}, "Start value (V)"=-1.0, "End value (V)"=2.0, "Channels 2"=[0, 20, 21, 22, 23], "Name"="lockin_slow"}, {"Amplitude (mod. signal unit)"=0.005, "Lockin on/off status"=FALSE, "Advanced options"={"Z-Controller Hold"=TRUE, "Record final Z"=FALSE, "Reset Bias"=TRUE}, "Backward sweep"=TRUE, "Number of points"=310, "Channels"=["Current (A)", "LI Demod 1 X (A)", "LI Demod 1 Y (A)", "LI Demod 2 X (A)", "LI Demod 2 Y (A)"], "Parameters"=["X (m)", "Y (m)", "Z (m)", "Z offset (m)", "Settling time (s)", "Integration time (s)", "Z-Ctrl hold", "Final Z (m)"], "Fixed parameters"=["Sweep Start", "Sweep End"], "Multiple sweeps configuration"={"Number of Sweeps"=2, "Save all"=FALSE}, "Initialization"={"Z averaging time (s)"=0.001, "Z offset (m)"=0.0, "Initial settling time (s)"=0.0031}, "Sweep Timing"={"Max. slew rate (V/s)"=inf, "Settling time (s)"=0.0031, "Integration time (s)"=0.0246}, "End of Sweep"={"End settling time (s)"=5e-05, "Z control time (s)"=5e-05}, "Start value (V)"=1.5, "End value (V)"=-0.05, "Channels 2"=[0, 20, 21, 22, 23], "Name"="Lock_in_DCA_1.5V->-50mV"}, {"Amplitude (mod. signal unit)"=0.005, "Lockin on/off status"=FALSE, "Advanced options"={"Z-Controller Hold"=TRUE, "Record final Z"=FALSE, "Reset Bias"=TRUE}, "Backward sweep"=TRUE, "Number of points"=401, "Channels"=["Current (A)", "Z (m)", "LI Demod 1 X (A)", "LI Demod 1 Y (A)", "LI Demod 2 X (A)", "LI Demod 2 Y (A)"], "Parameters"=["X (m)", "Y (m)", "Z (m)", "Z offset (m)", "Settling time (s)", "Integration time (s)", "Z-Ctrl hold", "Final Z (m)"], "Fixed parameters"=["Sweep Start", "Sweep End"], "Multiple sweeps configuration"={"Number of Sweeps"=1, "Save all"=FALSE}, "Initialization"={"Z averaging time (s)"=0.001, "Z offset (m)"=0.0, "Initial settling time (s)"=0.004}, "Sweep Timing"={"Max. slew rate (V/s)"=inf, "Settling time (s)"=0.02, "Integration time (s)"=0.015}, "End of Sweep"={"End settling time (s)"=5e-05, "Z control time (s)"=0.001}, "Start value (V)"=-1.0, "End value (V)"=1.0, "Channels 2"=[0, 14, 20, 21, 22, 23], "Name"="Long_MgPc_lockin_-1->1V"}, {"Amplitude (mod. signal unit)"=0.005, "Lockin on/off status"=FALSE, "Advanced options"={"Z-Controller Hold"=TRUE, "Record final Z"=FALSE, "Reset Bias"=TRUE}, "Backward sweep"=TRUE, "Number of points"=467, "Channels"=["Current (A)", "Z (m)", "LI Demod 1 X (A)", "LI Demod 1 Y (A)", "LI Demod 2 X (A)", "LI Demod 2 Y (A)"], "Parameters"=["X (m)", "Y (m)", "Z (m)", "Z offset (m)", "Settling time (s)", "Integration time (s)", "Z-Ctrl hold", "Final Z (m)"], "Fixed parameters"=["Sweep Start", "Sweep End"], "Multiple sweeps configuration"={"Number of Sweeps"=2, "Save all"=FALSE}, "Initialization"={"Z averaging time (s)"=0.001, "Z offset (m)"=0.0, "Initial settling time (s)"=0.004}, "Sweep Timing"={"Max. slew rate (V/s)"=inf, "Settling time (s)"=0.02, "Integration time (s)"=0.0246}, "End of Sweep"={"End settling time (s)"=5e-05, "Z control time (s)"=0.001}, "Start value (V)"=-2.0, "End value (V)"=1.5, "Channels 2"=[0, 14, 20, 21, 22, 23], "Name"="MgPc_long_lockin"}, {"Amplitude (mod. signal unit)"=0.008, "Lockin on/off status"=FALSE, "Advanced options"={"Z-Controller Hold"=TRUE, "Record final Z"=FALSE, "Reset Bias"=TRUE}, "Backward sweep"=TRUE, "Number of points"=256, "Channels"=["Current (A)", "LI Demod 1 X (A)", "LI Demod 1 Y (A)", "LI Demod 2 X (A)", "LI Demod 2 Y (A)"], "Parameters"=["X (m)", "Y (m)", "Z (m)", "Z offset (m)", "Settling time (s)", "Integration time (s)", "Z-Ctrl hold", "Final Z (m)"], "Fixed parameters"=["Sweep Start", "Sweep End"], "Multiple sweeps configuration"={"Number of Sweeps"=3, "Save all"=FALSE}, "Initialization"={"Z averaging time (s)"=0.001, "Z offset (m)"=0.0, "Initial settling time (s)"=0.0033}, "Sweep Timing"={"Max. slew rate (V/s)"=inf, "Settling time (s)"=0.0033, "Integration time (s)"=0.0082}, "End of Sweep"={"End settling time (s)"=5e-05, "Z control time (s)"=5e-05}, "Start value (V)"=-1.0, "End value (V)"=2.0, "Channels 2"=[0, 20, 21, 22, 23], "Name"="lockin_slow_-1_2"}, {"Amplitude (mod. signal unit)"=0.008, "Lockin on/off status"=FALSE, "Advanced options"={"Z-Controller Hold"=TRUE, "Record final Z"=FALSE, "Reset Bias"=TRUE}, "Backward sweep"=TRUE, "Number of points"=421, "Channels"=["Current (A)", "Z (m)", "LI Demod 1 X (A)", "LI Demod 1 Y (A)", "LI Demod 2 X (A)", "LI Demod 2 Y (A)"], "Parameters"=["X (m)", "Y (m)", "Z (m)", "Z offset (m)", "Settling time (s)", "Integration time (s)", "Z-Ctrl hold", "Final Z (m)"], "Fixed parameters"=["Sweep Start", "Sweep End"], "Multiple sweeps configuration"={"Number of Sweeps"=2, "Save all"=FALSE}, "Initialization"={"Z averaging time (s)"=0.001, "Z offset (m)"=0.0, "Initial settling time (s)"=5e-05}, "Sweep Timing"={"Max. slew rate (V/s)"=inf, "Settling time (s)"=0.0164, "Integration time (s)"=0.0164}, "End of Sweep"={"End settling time (s)"=5e-05, "Z control time (s)"=0.001}, "Start value (V)"=-2.0, "End value (V)"=2.2, "Channels 2"=[0, 14, 20, 21, 22, 23], "Name"="MgPc_long_lockin2"}, {"Amplitude (mod. signal unit)"=0.01, "Lockin on/off status"=FALSE, "Advanced options"={"Z-Controller Hold"=TRUE, "Record final Z"=FALSE, "Reset Bias"=TRUE}, "Backward sweep"=TRUE, "Number of points"=512, "Channels"=["Current (A)", "LI Demod 1 X (A)", "LI Demod 1 Y (A)", "LI Demod 2 X (A)", "LI Demod 2 Y (A)"], "Parameters"=["X (m)", "Y (m)", "Z (m)", "Z offset (m)", "Settling time (s)", "Integration time (s)", "Z-Ctrl hold", "Final Z (m)"], "Fixed parameters"=["Sweep Start", "Sweep End"], "Multiple sweeps configuration"={"Number of Sweeps"=1, "Save all"=FALSE}, "Initialization"={"Z averaging time (s)"=0.001, "Z offset (m)"=0.0, "Initial settling time (s)"=0.2}, "Sweep Timing"={"Max. slew rate (V/s)"=inf, "Settling time (s)"=0.0082, "Integration time (s)"=0.041}, "End of Sweep"={"End settling time (s)"=5e-05, "Z control time (s)"=5e-05}, "Start value (V)"=-3.0, "End value (V)"=2.0, "Channels 2"=[0, 20, 21, 22, 23], "Name"="Quick_Lockin"}]
  in  "Save As":string
  in  "Zspecparam.txt location":path=path "D:/Scripts/STSparam - Copy (2).txt"
  in  "Save As 2":string
  in  "STSparam.txt location":path=path "D:/Scripts/STSparam.txt"
  in  "Update STS/Zspec Param List":bool
  in  "START EXPERIMENT":bool
  in  "stop":bool
  in  "Duplicate Page 1":bool
  in  "No. of Exp":dbl=2.0 caption="No. of Experiments \n(If more than 5, edit VI)" step=1.0
  in  "Tab Control":T3(tab)=enum."Page 2"
  in  "Experiment 1":T4={"Drift Correction Settings"={"Drift Correction every"=4, "Drift correction Pixels"=128, "Channel index (0-23)"=0, "MaxImagesBack"=2, "Threshold"=2, "Increment"=1, "max applied Drift Correction"=40, "Correct Drift"=TRUE, "Correlate"=0, "Correct z drift"=FALSE, "zdrift \nDuration (s)"=0.0}, "Spectroscopy Setting"={"Imaging Current"=5e-11, "ref Current"=5e-12, "tip Speed (m/s)"=2e-09, "Imaging Bias"=-2.4, "ref Bias"=-0.02, "preSTS delay [ms]"=500, "STS z offset"=2e-10, "during Spec Bias (V)"=-0.02, "trigger1 < Hz"=0.0, "trigger 2 >Hz"=0.0, "autoStop"=FALSE, "Spectroscopy"=0, "PLL ON/OFF"=FALSE, "readjust setpoint every "=1, "z Reference"=TRUE, "Lock In"=FALSE}, "Misc"={"File name"="DCA_Zdependence_STS_Neg_Bias_Mol5_1_zOffset=200pm", "Email when finished"="Dhaneesh.Gopalakrishnan@monash.edu"}, "Grid Settings"={"type"=0, "type order"=0, "X pixel"=6, "Y pixel"=1, "Grid_Parms"={"center X (m)"=0.0, "center Y (m)"=0.0, "width (m)"=0.0, "height (m)"=0.0, "angle (deg)"=0.0}}, "STS Param List #1 "=4, "ZSpec Param List #1  "=0, "Repeat Experiment"={"Repeat"=TRUE, "Repeat Parameter"=2, "Values List #1"=14}} {"Repeat Experiment"."Repeat Parameter" items=["ref Current", "ref Bias", "STS z offset", "during Spec Bias (V)"]; "STS Param List #1" items=["numerical_DCA_-20mV->-3V", "numerical_DCA_-20mV->0.7V", "numerical_DCA_-20mV->-3V_3sweeps", "numerical_DCA_-20mV->-0.7V_30sweeps", "numerical_DCA_-20mV->-3V_50sweeps", "numerical_DCA_-20mV->-0.7V_50_sweeps", "numerical_DCA_-20mV->-3V_70sweeps", "numerical_DCA_-20mV->3V_100_sweeps", "numerical_DCA_-1V_>-3.2V_10sweeps", "numerical_DCA_-1V_>-3.2V_50sweeps", "numerical_DCA_-200m->800mV_50sweeps", "numerical_-1V->2V", "numerical_-20mV->20mV", "numerical_DCA_150mV->400mV", "DCA_numerical_-0.2V->0.8V", "V_star4_-20mV->-3V_3sweeps", "numerical_DCA_-20mV->-3V_10sweeps", "V_star2_-20mV->-3V_3sweeps", "V_star3_-20mV->-3.2V_3sweeps", "V_star5_-20mV->-3.5V_35sweeps", "V_star1_-20mV->-3.5V_70sweeps", "numerical_DCA_-20mV->-0.7V_50_sweepsV2", "numerical_DCA_0.12V_>0.6V_50sweeps", "numerical_-2V->2.2V", "DCA_numerical2_-0.2V->0.8V", "numerical_DCA_-200m->800mV_50sweepsV2", "lockin_-20mV->20mV", "lockin_-25mV->25mV", "test", "lockin_highRes_20mV_-20mV", "lockin_slow", "Lock_in_DCA_1.5V->-50mV", "Long_MgPc_lockin_-1->1V", "MgPc_long_lockin", "lockin_slow_-1_2", "MgPc_long_lockin2", "Quick_Lockin"]; "Grid Settings"."type order" items=["Grid", "Random", "Adam7"]; "Grid Settings"."type" items=["Line", "Grid", "Cloud"]; "Spectroscopy Setting"."Spectroscopy" items=["Bias", "zSpec"]; "Spectroscopy Setting"."trigger 2 >Hz" format="%#_6p"; "Spectroscopy Setting"."trigger1 < Hz" format="%#_6p"; "Spectroscopy Setting"."during Spec Bias (V)" format="%#_5p"; "Spectroscopy Setting"."STS z offset" format="%#_6p"; "Spectroscopy Setting"."ref Bias" format="%#_6p"; "Spectroscopy Setting"."Imaging Bias" format="%#_6p"; "Spectroscopy Setting"."tip Speed (m/s)" format="%.2p"; "Spectroscopy Setting"."ref Current" format="%#_6p"; "Spectroscopy Setting"."Imaging Current" format="%#_6p"; "Drift Correction Settings"."Correlate" items=["first Frame", "successive Frames"]; "Drift Correction Settings"."max applied Drift Correction" min=1 max=100 step=1 format="%.0p"; "Drift Correction Settings"."Threshold" min=1 step=1; "Drift Correction Settings"."Channel index (0-23)" items=["Current"=0, "Z (m)"=14]}
  in  "Experiment 2":T5={"Drift Correction Settings"={"Drift Correction every"=1, "Drift correction Pixels"=128, "Channel index (0-23)"=0, "MaxImagesBack"=2, "Threshold"=2, "Increment"=1, "max applied Drift Correction"=40, "Correct Drift"=TRUE, "Correlate"=0, "Correct z drift"=FALSE, "zdrift \nDuration (s)"=0.0}, "Spectroscopy Setting"={"Imaging Current"=5e-11, "ref Current"=5e-12, "tip Speed (m/s)"=2e-09, "Imaging Bias"=-2.4, "ref Bias"=-0.02, "preSTS delay [ms]"=500, "STS z offset"=0.0, "during Spec Bias (V)"=-0.02, "trigger1 < Hz"=0.0, "trigger 2 >Hz"=0.0, "autoStop"=FALSE, "Spectroscopy"=0, "PLL ON/OFF"=FALSE, "readjust setpoint every "=1, "z Reference"=TRUE, "Lock In"=FALSE}, "Misc"={"File name"="DCA_Zdependence_STS_Neg_Bias_Mol5_1", "Email when finished"="Dhaneesh.Gopalakrishnan@monash.edu"}, "Grid Settings"={"type"=0, "type order"=0, "X pixel"=6, "Y pixel"=1, "Grid_Parms"={"center X (m)"=0.0, "center Y (m)"=0.0, "width (m)"=0.0, "height (m)"=0.0, "angle (deg)"=0.0}}, "STS Param List #2 "=0, "ZSpec Param List  #2 "=0, "Repeat Experiment"={"Repeat"=TRUE, "Repeat Parameter"=2, "Values List #2"=7}} {"Repeat Experiment"."Repeat Parameter" items=["ref Current", "ref Bias", "STS z offset", "during Spec Bias (V)"]; "STS Param List #2" items=["numerical_DCA_-20mV->-3V", "numerical_DCA_-20mV->0.7V", "numerical_DCA_-20mV->-3V_3sweeps", "numerical_DCA_-20mV->-0.7V_30sweeps", "numerical_DCA_-20mV->-3V_50sweeps", "numerical_DCA_-20mV->-0.7V_50_sweeps", "numerical_DCA_-20mV->-3V_70sweeps", "numerical_DCA_-20mV->3V_100_sweeps", "numerical_DCA_-1V_>-3.2V_10sweeps", "numerical_DCA_-1V_>-3.2V_50sweeps", "numerical_DCA_-200m->800mV_50sweeps", "numerical_-1V->2V", "numerical_-20mV->20mV", "numerical_DCA_150mV->400mV", "DCA_numerical_-0.2V->0.8V", "V_star4_-20mV->-3V_3sweeps", "numerical_DCA_-20mV->-3V_10sweeps", "V_star2_-20mV->-3V_3sweeps", "V_star3_-20mV->-3.2V_3sweeps", "V_star5_-20mV->-3.5V_35sweeps", "V_star1_-20mV->-3.5V_70sweeps", "numerical_DCA_-20mV->-0.7V_50_sweepsV2", "numerical_DCA_0.12V_>0.6V_50sweeps", "numerical_-2V->2.2V", "DCA_numerical2_-0.2V->0.8V", "numerical_DCA_-200m->800mV_50sweepsV2", "lockin_-20mV->20mV", "lockin_-25mV->25mV", "test", "lockin_highRes_20mV_-20mV", "lockin_slow", "Lock_in_DCA_1.5V->-50mV", "Long_MgPc_lockin_-1->1V", "MgPc_long_lockin", "lockin_slow_-1_2", "MgPc_long_lockin2", "Quick_Lockin"]; "Grid Settings"."type order" items=["Grid", "Random", "Adam7"]; "Grid Settings"."type" items=["Line", "Grid", "Cloud"]; "Spectroscopy Setting"."Spectroscopy" items=["Bias", "zSpec"]; "Spectroscopy Setting"."trigger 2 >Hz" format="%#_6p"; "Spectroscopy Setting"."trigger1 < Hz" format="%#_6p"; "Spectroscopy Setting"."during Spec Bias (V)" format="%#_5p"; "Spectroscopy Setting"."STS z offset" format="%#_6p"; "Spectroscopy Setting"."ref Bias" format="%#_6p"; "Spectroscopy Setting"."Imaging Bias" format="%#_6p"; "Spectroscopy Setting"."tip Speed (m/s)" format="%.2p"; "Spectroscopy Setting"."ref Current" format="%#_6p"; "Spectroscopy Setting"."Imaging Current" format="%#_6p"; "Drift Correction Settings"."Correlate" items=["first Frame", "successive Frames"]; "Drift Correction Settings"."max applied Drift Correction" min=1 max=100 step=1 format="%.0p"; "Drift Correction Settings"."Threshold" min=1 step=1; "Drift Correction Settings"."Channel index (0-23)" items=["Current"=0, "Z (m)"=14]}
  in  "Experiment 3":T6={"Drift Correction Settings"={"Drift Correction every"=6, "Drift correction Pixels"=128, "Channel index (0-23)"=0, "MaxImagesBack"=2, "Threshold"=2, "Increment"=1, "max applied Drift Correction"=40, "Correct Drift"=TRUE, "Correlate"=0, "Correct z drift"=FALSE, "zdrift \nDuration (s)"=0.0}, "Spectroscopy Setting"={"Imaging Current"=5e-11, "ref Current"=5e-12, "tip Speed (m/s)"=2e-09, "Imaging Bias"=-2.4, "ref Bias"=-0.02, "preSTS delay [ms]"=500, "STS z offset"=4e-10, "during Spec Bias (V)"=-0.02, "trigger1 < Hz"=0.0, "trigger 2 >Hz"=0.0, "autoStop"=FALSE, "Spectroscopy"=0, "PLL ON/OFF"=FALSE, "readjust setpoint every "=1, "z Reference"=TRUE, "Lock In"=FALSE}, "Misc"={"File name"="DCA_Zdependence_STS_Neg_Bias_Mol5_1", "Email when finished"="Dhaneesh.Gopalakrishnan@monash.edu"}, "Grid Settings"={"type"=0, "type order"=0, "X pixel"=6, "Y pixel"=1, "Grid_Parms"={"center X (m)"=0.0, "center Y (m)"=0.0, "width (m)"=0.0, "height (m)"=0.0, "angle (deg)"=0.0}}, "STS Param List #3 "=4, "ZSpec Param List #3 "=0, "Repeat Experiment"={"Repeat"=TRUE, "Repeat Parameter"=2, "Values List #3"=7}} {"Repeat Experiment"."Repeat Parameter" items=["ref Current", "ref Bias", "STS z offset", "during Spec Bias (V)"]; "STS Param List #3" items=["numerical_DCA_-20mV->-3V", "numerical_DCA_-20mV->0.7V", "numerical_DCA_-20mV->-3V_3sweeps", "numerical_DCA_-20mV->-0.7V_30sweeps", "numerical_DCA_-20mV->-3V_50sweeps", "numerical_DCA_-20mV->-0.7V_50_sweeps", "numerical_DCA_-20mV->-3V_70sweeps", "numerical_DCA_-20mV->3V_100_sweeps", "numerical_DCA_-1V_>-3.2V_10sweeps", "numerical_DCA_-1V_>-3.2V_50sweeps", "numerical_DCA_-200m->800mV_50sweeps", "numerical_-1V->2V", "numerical_-20mV->20mV", "numerical_DCA_150mV->400mV", "DCA_numerical_-0.2V->0.8V", "V_star4_-20mV->-3V_3sweeps", "numerical_DCA_-20mV->-3V_10sweeps", "V_star2_-20mV->-3V_3sweeps", "V_star3_-20mV->-3.2V_3sweeps", "V_star5_-20mV->-3.5V_35sweeps", "V_star1_-20mV->-3.5V_70sweeps", "numerical_DCA_-20mV->-0.7V_50_sweepsV2", "numerical_DCA_0.12V_>0.6V_50sweeps", "numerical_-2V->2.2V", "DCA_numerical2_-0.2V->0.8V", "numerical_DCA_-200m->800mV_50sweepsV2", "lockin_-20mV->20mV", "lockin_-25mV->25mV", "test", "lockin_highRes_20mV_-20mV", "lockin_slow", "Lock_in_DCA_1.5V->-50mV", "Long_MgPc_lockin_-1->1V", "MgPc_long_lockin", "lockin_slow_-1_2", "MgPc_long_lockin2", "Quick_Lockin"]; "Grid Settings"."type order" items=["Grid", "Random", "Adam7"]; "Grid Settings"."type" items=["Line", "Grid", "Cloud"]; "Spectroscopy Setting"."Spectroscopy" items=["Bias", "zSpec"]; "Spectroscopy Setting"."trigger 2 >Hz" format="%#_6p"; "Spectroscopy Setting"."trigger1 < Hz" format="%#_6p"; "Spectroscopy Setting"."during Spec Bias (V)" format="%#_5p"; "Spectroscopy Setting"."STS z offset" format="%#_6p"; "Spectroscopy Setting"."ref Bias" format="%#_6p"; "Spectroscopy Setting"."Imaging Bias" format="%#_6p"; "Spectroscopy Setting"."tip Speed (m/s)" format="%.2p"; "Spectroscopy Setting"."ref Current" format="%#_6p"; "Spectroscopy Setting"."Imaging Current" format="%#_6p"; "Drift Correction Settings"."Correlate" items=["first Frame", "successive Frames"]; "Drift Correction Settings"."max applied Drift Correction" min=1 max=100 step=1 format="%.0p"; "Drift Correction Settings"."Threshold" min=1 step=1; "Drift Correction Settings"."Channel index (0-23)" items=["Current"=0, "Z (m)"=14]}
  in  "Experiment 4":T7={"Drift Correction Settings"={"Drift Correction every"=1, "Drift correction Pixels"=128, "Channel index (0-23)"=0, "MaxImagesBack"=2, "Threshold"=2, "Increment"=1, "max applied Drift Correction"=40, "Correct Drift"=TRUE, "Correlate"=0, "Correct z drift"=FALSE, "zdrift \nDuration (s)"=0.0}, "Spectroscopy Setting"={"Imaging Current"=5e-11, "ref Current"=5e-12, "tip Speed (m/s)"=1e-08, "Imaging Bias"=-2.4, "ref Bias"=-0.02, "preSTS delay [ms]"=500, "STS z offset"=0.0, "during Spec Bias (V)"=-0.02, "trigger1 < Hz"=0.0, "trigger 2 >Hz"=0.0, "autoStop"=FALSE, "Spectroscopy"=0, "PLL ON/OFF"=FALSE, "readjust setpoint every "=1, "z Reference"=TRUE, "Lock In"=FALSE}, "Misc"={"File name"="DCA_Zdependence_STS_Neg_Bias_Mol5_1", "Email when finished"="Dhaneesh.Gopalakrishnan@monash.edu"}, "Grid Settings"={"type"=0, "type order"=0, "X pixel"=6, "Y pixel"=1, "Grid_Parms"={"center X (m)"=0.0, "center Y (m)"=0.0, "width (m)"=0.0, "height (m)"=0.0, "angle (deg)"=0.0}}, "STS Param List #4 "=0, "ZSpec Param List  #4"=0, "Repeat Experiment"={"Repeat"=TRUE, "Repeat Parameter"=2, "Values List #4"=7}} {"Repeat Experiment"."Repeat Parameter" items=["ref Current", "ref Bias", "STS z offset", "during Spec Bias (V)"]; "STS Param List #4" items=["numerical_DCA_-20mV->-3V", "numerical_DCA_-20mV->0.7V", "numerical_DCA_-20mV->-3V_3sweeps", "numerical_DCA_-20mV->-0.7V_30sweeps", "numerical_DCA_-20mV->-3V_50sweeps", "numerical_DCA_-20mV->-0.7V_50_sweeps", "numerical_DCA_-20mV->-3V_70sweeps", "numerical_DCA_-20mV->3V_100_sweeps", "numerical_DCA_-1V_>-3.2V_10sweeps", "numerical_DCA_-1V_>-3.2V_50sweeps", "numerical_DCA_-200m->800mV_50sweeps", "numerical_-1V->2V", "numerical_-20mV->20mV", "numerical_DCA_150mV->400mV", "DCA_numerical_-0.2V->0.8V", "V_star4_-20mV->-3V_3sweeps", "numerical_DCA_-20mV->-3V_10sweeps", "V_star2_-20mV->-3V_3sweeps", "V_star3_-20mV->-3.2V_3sweeps", "V_star5_-20mV->-3.5V_35sweeps", "V_star1_-20mV->-3.5V_70sweeps", "numerical_DCA_-20mV->-0.7V_50_sweepsV2", "numerical_DCA_0.12V_>0.6V_50sweeps", "numerical_-2V->2.2V", "DCA_numerical2_-0.2V->0.8V", "numerical_DCA_-200m->800mV_50sweepsV2", "lockin_-20mV->20mV", "lockin_-25mV->25mV", "test", "lockin_highRes_20mV_-20mV", "lockin_slow", "Lock_in_DCA_1.5V->-50mV", "Long_MgPc_lockin_-1->1V", "MgPc_long_lockin", "lockin_slow_-1_2", "MgPc_long_lockin2", "Quick_Lockin"]; "Grid Settings"."type order" items=["Grid", "Random", "Adam7"]; "Grid Settings"."type" items=["Line", "Grid", "Cloud"]; "Spectroscopy Setting"."Spectroscopy" items=["Bias", "zSpec"]; "Spectroscopy Setting"."trigger 2 >Hz" format="%#_6p"; "Spectroscopy Setting"."trigger1 < Hz" format="%#_6p"; "Spectroscopy Setting"."during Spec Bias (V)" format="%#_5p"; "Spectroscopy Setting"."STS z offset" format="%#_6p"; "Spectroscopy Setting"."ref Bias" format="%#_6p"; "Spectroscopy Setting"."Imaging Bias" format="%#_6p"; "Spectroscopy Setting"."tip Speed (m/s)" format="%.2p"; "Spectroscopy Setting"."ref Current" format="%#_6p"; "Spectroscopy Setting"."Imaging Current" format="%#_6p"; "Drift Correction Settings"."Correlate" items=["first Frame", "successive Frames"]; "Drift Correction Settings"."max applied Drift Correction" min=1 max=100 step=1 format="%.0p"; "Drift Correction Settings"."Threshold" min=1 step=1; "Drift Correction Settings"."Channel index (0-23)" items=["Current"=0, "Z (m)"=14]}
  in  "Experiment 5":T8={"Drift Correction Settings"={"Drift Correction every"=1, "Drift correction Pixels"=256, "Channel index (0-23)"=0, "MaxImagesBack"=2, "Threshold"=2, "Increment"=1, "max applied Drift Correction"=40, "Correct Drift"=TRUE, "Correlate"=0, "Correct z drift"=FALSE, "zdrift \nDuration (s)"=0.0}, "Spectroscopy Setting"={"Imaging Current"=5e-11, "ref Current"=5e-12, "tip Speed (m/s)"=1e-08, "Imaging Bias"=-2.4, "ref Bias"=-0.02, "preSTS delay [ms]"=500, "STS z offset"=0.0, "during Spec Bias (V)"=-0.02, "trigger1 < Hz"=0.0, "trigger 2 >Hz"=0.0, "autoStop"=FALSE, "Spectroscopy"=0, "PLL ON/OFF"=FALSE, "readjust setpoint every "=1, "z Reference"=TRUE, "Lock In"=FALSE}, "Misc"={"File name"="DCA_Zdependence_STS_Pos_Bias_Mol9_46", "Email when finished"="Dhaneesh.Gopalakrishnan@monash.edu"}, "Grid Settings"={"type"=0, "type order"=0, "X pixel"=27, "Y pixel"=1, "Grid_Parms"={"center X (m)"=0.0, "center Y (m)"=0.0, "width (m)"=0.0, "height (m)"=0.0, "angle (deg)"=0.0}}, "STS Param List #5 "=0, "ZSpec Param List #5  "=0, "Repeat Experiment"={"Repeat"=TRUE, "Repeat Parameter"=2, "Values List #5"=7}} {"Repeat Experiment"."Repeat Parameter" items=["ref Current", "ref Bias", "STS z offset", "during Spec Bias (V)"]; "STS Param List #5" items=["numerical_DCA_-20mV->-3V", "numerical_DCA_-20mV->0.7V", "numerical_DCA_-20mV->-3V_3sweeps", "numerical_DCA_-20mV->-0.7V_30sweeps", "numerical_DCA_-20mV->-3V_50sweeps", "numerical_DCA_-20mV->-0.7V_50_sweeps", "numerical_DCA_-20mV->-3V_70sweeps", "numerical_DCA_-20mV->3V_100_sweeps", "numerical_DCA_-1V_>-3.2V_10sweeps", "numerical_DCA_-1V_>-3.2V_50sweeps", "numerical_DCA_-200m->800mV_50sweeps", "numerical_-1V->2V", "numerical_-20mV->20mV", "numerical_DCA_150mV->400mV", "DCA_numerical_-0.2V->0.8V", "V_star4_-20mV->-3V_3sweeps", "numerical_DCA_-20mV->-3V_10sweeps", "V_star2_-20mV->-3V_3sweeps", "V_star3_-20mV->-3.2V_3sweeps", "V_star5_-20mV->-3.5V_35sweeps", "V_star1_-20mV->-3.5V_70sweeps", "numerical_DCA_-20mV->-0.7V_50_sweepsV2", "numerical_DCA_0.12V_>0.6V_50sweeps", "numerical_-2V->2.2V", "DCA_numerical2_-0.2V->0.8V", "numerical_DCA_-200m->800mV_50sweepsV2", "lockin_-20mV->20mV", "lockin_-25mV->25mV", "test", "lockin_highRes_20mV_-20mV", "lockin_slow", "Lock_in_DCA_1.5V->-50mV", "Long_MgPc_lockin_-1->1V", "MgPc_long_lockin", "lockin_slow_-1_2", "MgPc_long_lockin2", "Quick_Lockin"]; "Grid Settings"."type order" items=["Grid", "Random", "Adam7"]; "Grid Settings"."type" items=["Line", "Grid", "Cloud"]; "Spectroscopy Setting"."Spectroscopy" items=["Bias", "zSpec"]; "Spectroscopy Setting"."trigger 2 >Hz" format="%#_6p"; "Spectroscopy Setting"."trigger1 < Hz" format="%#_6p"; "Spectroscopy Setting"."during Spec Bias (V)" format="%#_5p"; "Spectroscopy Setting"."STS z offset" format="%#_6p"; "Spectroscopy Setting"."ref Bias" format="%#_6p"; "Spectroscopy Setting"."Imaging Bias" format="%#_6p"; "Spectroscopy Setting"."tip Speed (m/s)" format="%.2p"; "Spectroscopy Setting"."ref Current" format="%#_6p"; "Spectroscopy Setting"."Imaging Current" format="%#_6p"; "Drift Correction Settings"."Correlate" items=["first Frame", "successive Frames"]; "Drift Correction Settings"."max applied Drift Correction" min=1 max=100 step=1 format="%.0p"; "Drift Correction Settings"."Threshold" min=1 step=1; "Drift Correction Settings"."Channel index (0-23)" items=["Current"=0, "Z (m)"=14]}
  # "z Spectroscopy"
  # "GRID points"
  # "Increase this if no Drift was detected for \na certain number of images"
  # "% of image size"
  # "Only first frame works"
  # "z Spectroscopy"
  # "GRID points"
  # "Increase this if no Drift was detected for \na certain number of images"
  # "% of image size"
  # "Only first frame works"
  # "z Spectroscopy"
  # "GRID points"
  # "Increase this if no Drift was detected for \na certain number of images"
  # "% of image size"
  # "Only first frame works"
  # "z Spectroscopy"
  # "GRID points"
  # "Increase this if no Drift was detected for \na certain number of images"
  # "% of image size"
  # "Only first frame works"
  # "z Spectroscopy"
  # "GRID points"
  # "Increase this if no Drift was detected for \na certain number of images"
  # "% of image size"
  # "Only first frame works"
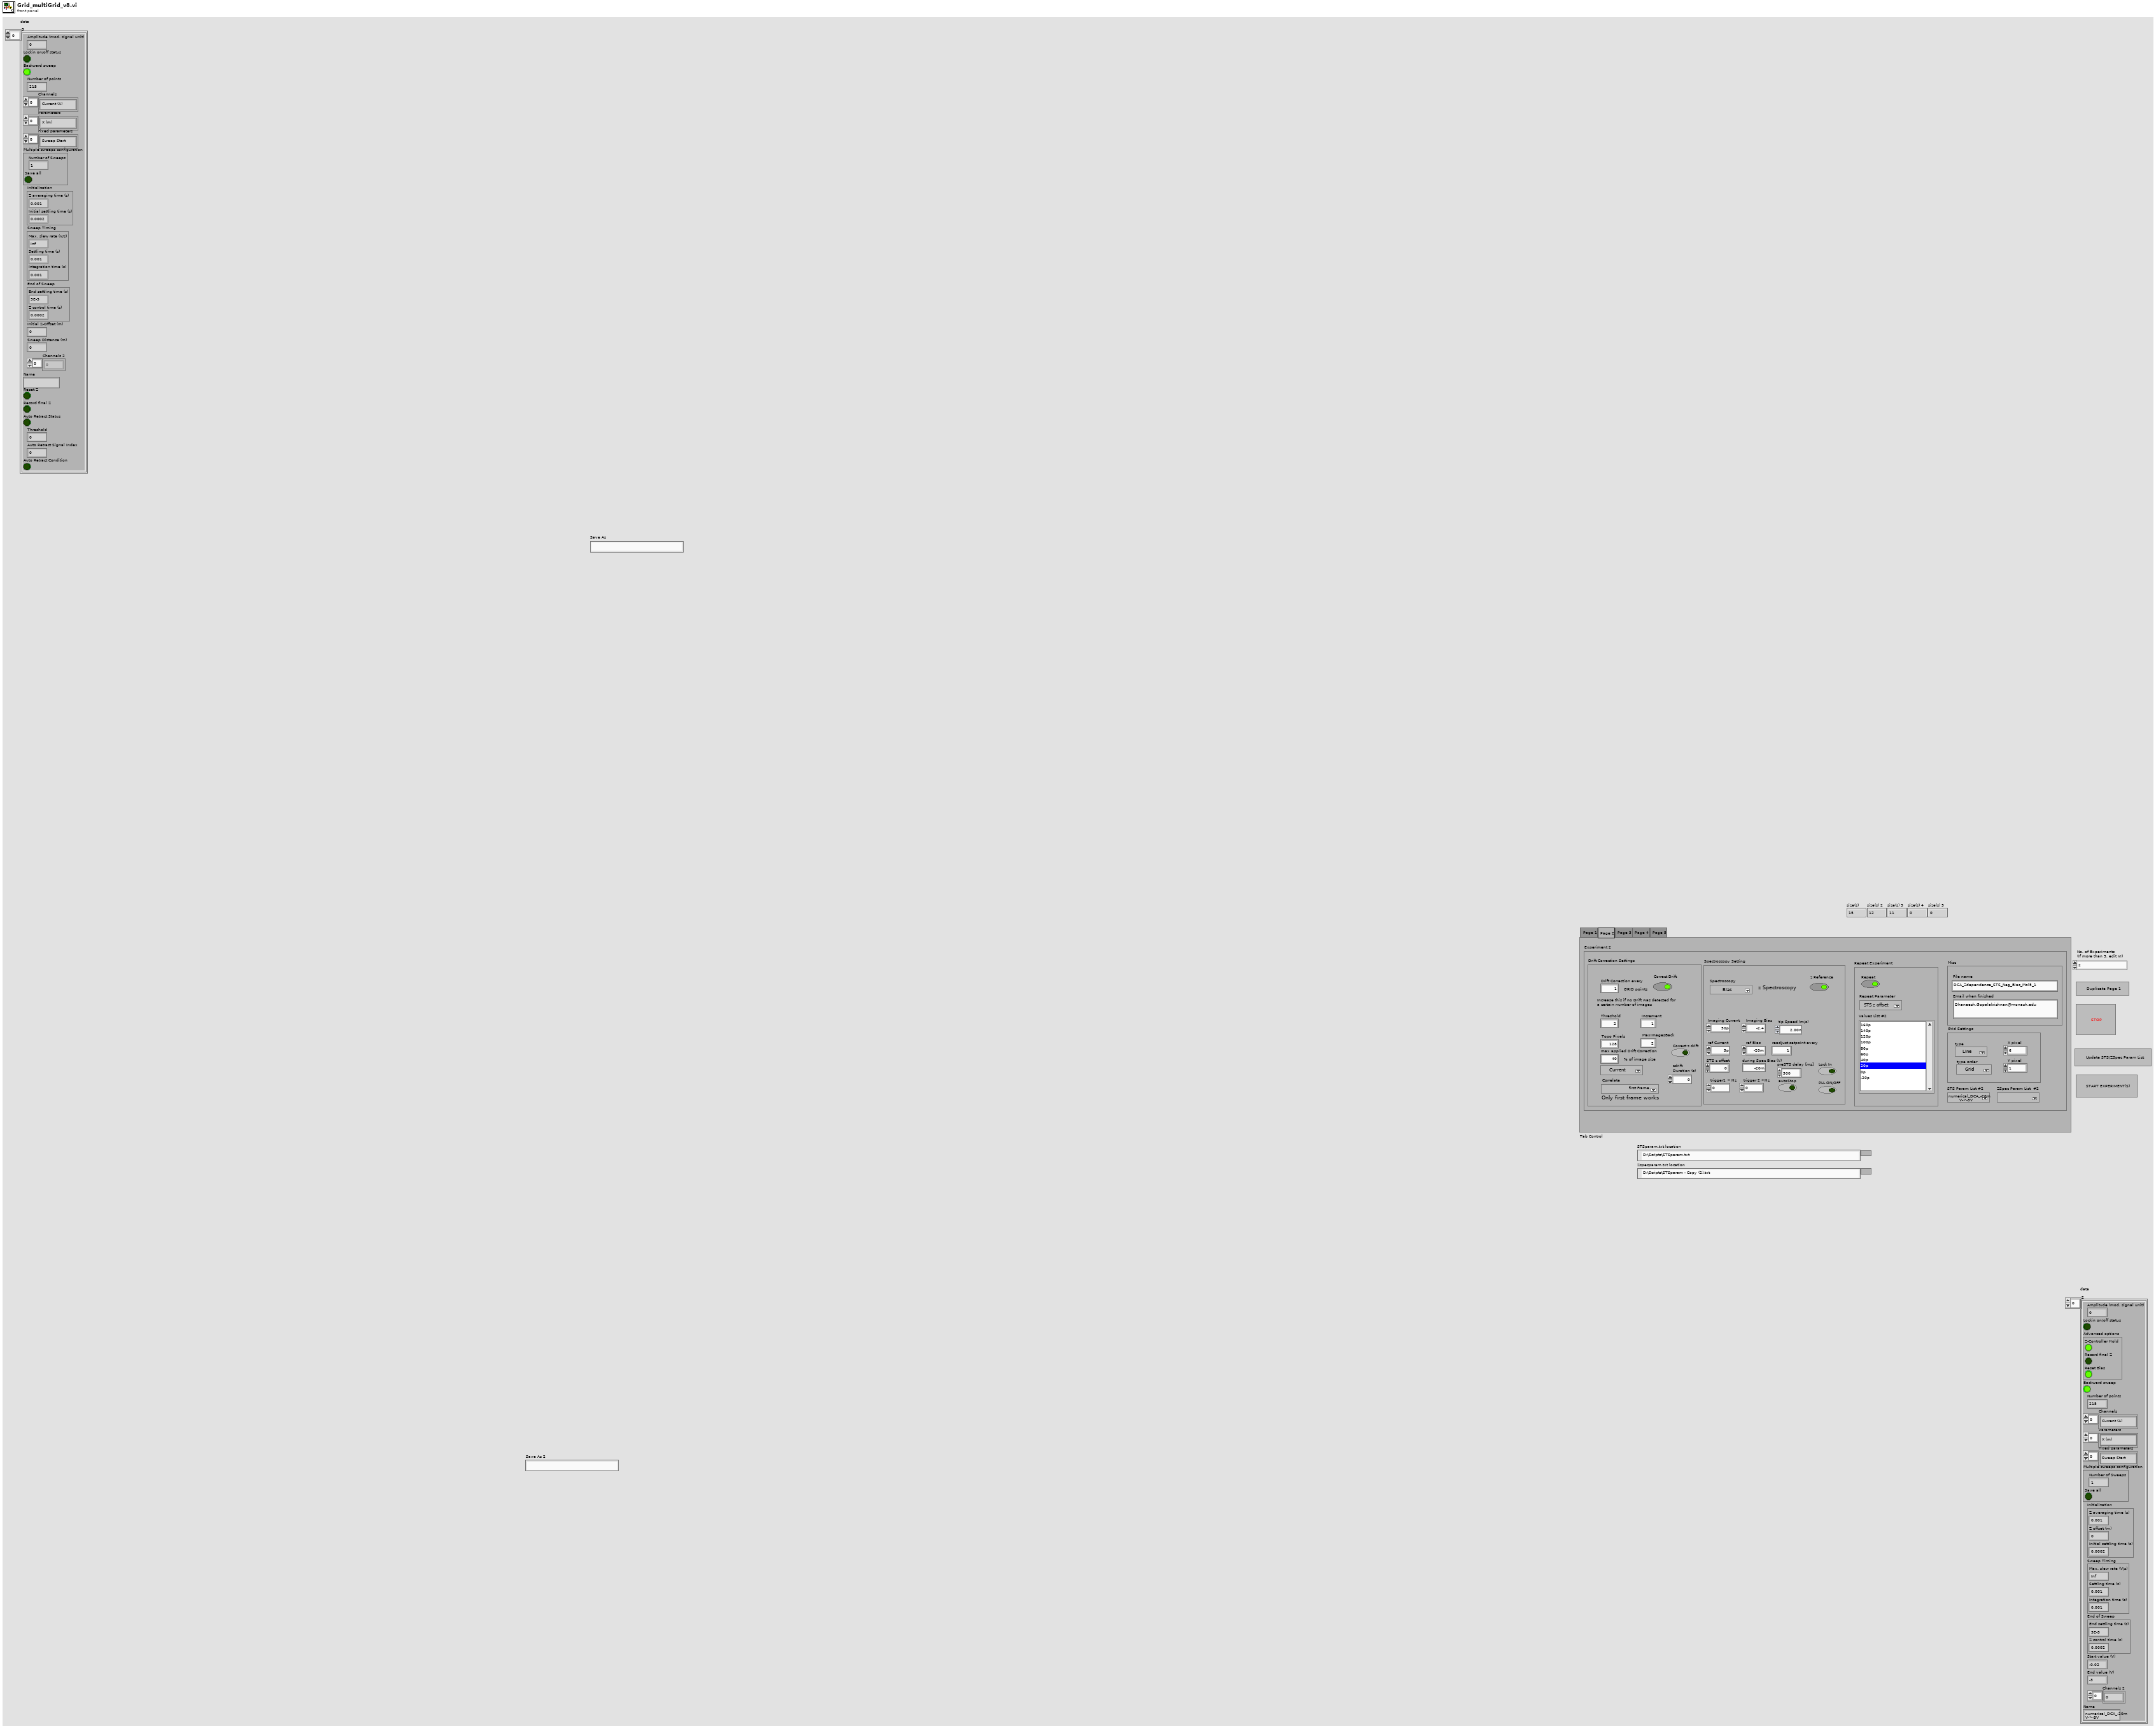
[diagram p1: front panel]
types:
  T1 = cluster{"Amplitude (mod. signal unit)":sgl, "Lockin on/off status":bool, "Backward sweep":bool, "Number of points":i32, "Channels":string[], "Parameters":string[], "Fixed parameters":string[], "Multiple sweeps configuration":cluster{"Number of Sweeps":i32, "Save all":bool}, "Initialization":cluster{"Z averaging time (s)":sgl, "Initial settling time (s)":sgl}, "Sweep Timing":cluster{"Max. slew rate (V/s)":sgl, "Settling time (s)":sgl, "Integration time (s)":sgl}, "End of Sweep":cluster{"End settling time (s)":sgl, "Z control time (s)":sgl}, "Initial Z-Offset (m)":sgl, "Sweep Distance (m)":sgl, "Channels 2":i32[], "Name":string, "Reset Z":bool, "Record final Z":bool, "Auto Retract Status":bool, "Threshold":sgl, "Auto Retract Signal Index":i32, "Auto Retract Condition":bool}[]
  T2 = cluster{"Amplitude (mod. signal unit)":sgl, "Lockin on/off status":bool, "Advanced options":cluster{"Z-Controller Hold":bool, "Record final Z":bool, "Reset Bias":bool}, "Backward sweep":bool, "Number of points":i32, "Channels":string[], "Parameters":string[], "Fixed parameters":string[], "Multiple sweeps configuration":cluster{"Number of Sweeps":i32, "Save all":bool}, "Initialization":cluster{"Z averaging time (s)":sgl, "Z offset (m)":sgl, "Initial settling time (s)":sgl}, "Sweep Timing":cluster{"Max. slew rate (V/s)":sgl, "Settling time (s)":sgl, "Integration time (s)":sgl}, "End of Sweep":cluster{"End settling time (s)":sgl, "Z control time (s)":sgl}, "Start value (V)":sgl, "End value (V)":sgl, "Channels 2":i32[], "Name":string}[]
  T3 = enum32{"Page 1", "Page 2", "Page 3", "Page 4", "Page 5"}
  T4 = cluster{"Drift Correction Settings":cluster{"Drift Correction every":i32, "Drift correction Pixels":i32, "Channel index (0-23)":u8, "MaxImagesBack":i32, "Threshold":i32, "Increment":i32, "max applied Drift Correction":i32, "Correct Drift":bool, "Correlate":u16, "Correct z drift":bool, "zdrift \nDuration (s)":dbl}, "Spectroscopy Setting":cluster{"Imaging Current":dbl, "ref Current":dbl, "tip Speed (m/s)":sgl, "Imaging Bias":dbl, "ref Bias":dbl, "preSTS delay [ms]":u32, "STS z offset":dbl, "during Spec Bias (V)":sgl, "trigger1 < Hz":sgl, "trigger 2 >Hz":sgl, "autoStop":bool, "Spectroscopy":u16, "PLL ON/OFF":bool, "readjust setpoint every ":i32, "z Reference":bool, "Lock In":bool}, "Misc":cluster{"File name":string, "Email when finished":string}, "Grid Settings":cluster{"type":u16, "type order":u16, "X pixel":i32, "Y pixel":i32, "Grid_Parms":cluster{"center X (m)":sgl, "center Y (m)":sgl, "width (m)":sgl, "height (m)":sgl, "angle (deg)":sgl}}, "STS Param List #1 ":u16, "ZSpec Param List #1  ":u16, "Repeat Experiment":cluster{"Repeat":bool, "Repeat Parameter":u16, "Values List #1":i32}}
  T5 = cluster{"Drift Correction Settings":cluster{"Drift Correction every":i32, "Drift correction Pixels":i32, "Channel index (0-23)":u8, "MaxImagesBack":i32, "Threshold":i32, "Increment":i32, "max applied Drift Correction":i32, "Correct Drift":bool, "Correlate":u16, "Correct z drift":bool, "zdrift \nDuration (s)":dbl}, "Spectroscopy Setting":cluster{"Imaging Current":dbl, "ref Current":dbl, "tip Speed (m/s)":sgl, "Imaging Bias":dbl, "ref Bias":dbl, "preSTS delay [ms]":u32, "STS z offset":dbl, "during Spec Bias (V)":sgl, "trigger1 < Hz":sgl, "trigger 2 >Hz":sgl, "autoStop":bool, "Spectroscopy":u16, "PLL ON/OFF":bool, "readjust setpoint every ":i32, "z Reference":bool, "Lock In":bool}, "Misc":cluster{"File name":string, "Email when finished":string}, "Grid Settings":cluster{"type":u16, "type order":u16, "X pixel":i32, "Y pixel":i32, "Grid_Parms":cluster{"center X (m)":sgl, "center Y (m)":sgl, "width (m)":sgl, "height (m)":sgl, "angle (deg)":sgl}}, "STS Param List #2 ":u16, "ZSpec Param List  #2 ":u16, "Repeat Experiment":cluster{"Repeat":bool, "Repeat Parameter":u16, "Values List #2":i32}}
  T6 = cluster{"Drift Correction Settings":cluster{"Drift Correction every":i32, "Drift correction Pixels":i32, "Channel index (0-23)":u8, "MaxImagesBack":i32, "Threshold":i32, "Increment":i32, "max applied Drift Correction":i32, "Correct Drift":bool, "Correlate":u16, "Correct z drift":bool, "zdrift \nDuration (s)":dbl}, "Spectroscopy Setting":cluster{"Imaging Current":dbl, "ref Current":dbl, "tip Speed (m/s)":sgl, "Imaging Bias":dbl, "ref Bias":dbl, "preSTS delay [ms]":u32, "STS z offset":dbl, "during Spec Bias (V)":sgl, "trigger1 < Hz":sgl, "trigger 2 >Hz":sgl, "autoStop":bool, "Spectroscopy":u16, "PLL ON/OFF":bool, "readjust setpoint every ":i32, "z Reference":bool, "Lock In":bool}, "Misc":cluster{"File name":string, "Email when finished":string}, "Grid Settings":cluster{"type":u16, "type order":u16, "X pixel":i32, "Y pixel":i32, "Grid_Parms":cluster{"center X (m)":sgl, "center Y (m)":sgl, "width (m)":sgl, "height (m)":sgl, "angle (deg)":sgl}}, "STS Param List #3 ":u16, "ZSpec Param List #3 ":u16, "Repeat Experiment":cluster{"Repeat":bool, "Repeat Parameter":u16, "Values List #3":i32}}
  T7 = cluster{"Drift Correction Settings":cluster{"Drift Correction every":i32, "Drift correction Pixels":i32, "Channel index (0-23)":u8, "MaxImagesBack":i32, "Threshold":i32, "Increment":i32, "max applied Drift Correction":i32, "Correct Drift":bool, "Correlate":u16, "Correct z drift":bool, "zdrift \nDuration (s)":dbl}, "Spectroscopy Setting":cluster{"Imaging Current":dbl, "ref Current":dbl, "tip Speed (m/s)":sgl, "Imaging Bias":dbl, "ref Bias":dbl, "preSTS delay [ms]":u32, "STS z offset":dbl, "during Spec Bias (V)":sgl, "trigger1 < Hz":sgl, "trigger 2 >Hz":sgl, "autoStop":bool, "Spectroscopy":u16, "PLL ON/OFF":bool, "readjust setpoint every ":i32, "z Reference":bool, "Lock In":bool}, "Misc":cluster{"File name":string, "Email when finished":string}, "Grid Settings":cluster{"type":u16, "type order":u16, "X pixel":i32, "Y pixel":i32, "Grid_Parms":cluster{"center X (m)":sgl, "center Y (m)":sgl, "width (m)":sgl, "height (m)":sgl, "angle (deg)":sgl}}, "STS Param List #4 ":u16, "ZSpec Param List  #4":u16, "Repeat Experiment":cluster{"Repeat":bool, "Repeat Parameter":u16, "Values List #4":i32}}
  T8 = cluster{"Drift Correction Settings":cluster{"Drift Correction every":i32, "Drift correction Pixels":i32, "Channel index (0-23)":u8, "MaxImagesBack":i32, "Threshold":i32, "Increment":i32, "max applied Drift Correction":i32, "Correct Drift":bool, "Correlate":u16, "Correct z drift":bool, "zdrift \nDuration (s)":dbl}, "Spectroscopy Setting":cluster{"Imaging Current":dbl, "ref Current":dbl, "tip Speed (m/s)":sgl, "Imaging Bias":dbl, "ref Bias":dbl, "preSTS delay [ms]":u32, "STS z offset":dbl, "during Spec Bias (V)":sgl, "trigger1 < Hz":sgl, "trigger 2 >Hz":sgl, "autoStop":bool, "Spectroscopy":u16, "PLL ON/OFF":bool, "readjust setpoint every ":i32, "z Reference":bool, "Lock In":bool}, "Misc":cluster{"File name":string, "Email when finished":string}, "Grid Settings":cluster{"type":u16, "type order":u16, "X pixel":i32, "Y pixel":i32, "Grid_Parms":cluster{"center X (m)":sgl, "center Y (m)":sgl, "width (m)":sgl, "height (m)":sgl, "angle (deg)":sgl}}, "STS Param List #5 ":u16, "ZSpec Param List #5  ":u16, "Repeat Experiment":cluster{"Repeat":bool, "Repeat Parameter":u16, "Values List #5":i32}}
  T9 = cluster{"Amplitude (mod. signal unit)":sgl, "Lockin on/off status":bool, "Backward sweep":bool, "Number of points":i32, "Channels":string[], "Parameters":string[], "Fixed parameters":string[], "Multiple sweeps configuration":cluster{"Number of Sweeps":i32, "Save all":bool}, "Initialization":cluster{"Z averaging time (s)":sgl, "Initial settling time (s)":sgl}, "Sweep Timing":cluster{"Max. slew rate (V/s)":sgl, "Settling time (s)":sgl, "Integration time (s)":sgl}, "End of Sweep":cluster{"End settling time (s)":sgl, "Z control time (s)":sgl}, "Initial Z-Offset (m)":sgl, "Sweep Distance (m)":sgl, "Channels 2":i32[], "Name":string, "Reset Z":bool, "Record final Z":bool, "Auto Retract Status":bool, "Threshold":sgl, "Auto Retract Signal Index":i32, "Auto Retract Condition":bool}
  T10 = cluster{"Amplitude (mod. signal unit)":sgl, "Lockin on/off status":bool, "Advanced options":cluster{"Z-Controller Hold":bool, "Record final Z":bool, "Reset Bias":bool}, "Backward sweep":bool, "Number of points":i32, "Channels":string[], "Parameters":string[], "Fixed parameters":string[], "Multiple sweeps configuration":cluster{"Number of Sweeps":i32, "Save all":bool}, "Initialization":cluster{"Z averaging time (s)":sgl, "Z offset (m)":sgl, "Initial settling time (s)":sgl}, "Sweep Timing":cluster{"Max. slew rate (V/s)":sgl, "Settling time (s)":sgl, "Integration time (s)":sgl}, "End of Sweep":cluster{"End settling time (s)":sgl, "Z control time (s)":sgl}, "Start value (V)":sgl, "End value (V)":sgl, "Channels 2":i32[], "Name":string}
  T11 = cluster{"Drift Correction every":i32, "Drift correction Pixels":i32, "Channel index (0-23)":u8, "MaxImagesBack":i32, "Threshold":i32, "Increment":i32, "max applied Drift Correction":i32, "Correct Drift":bool, "Correlate":u16, "Correct z drift":bool, "zdrift \nDuration (s)":dbl}
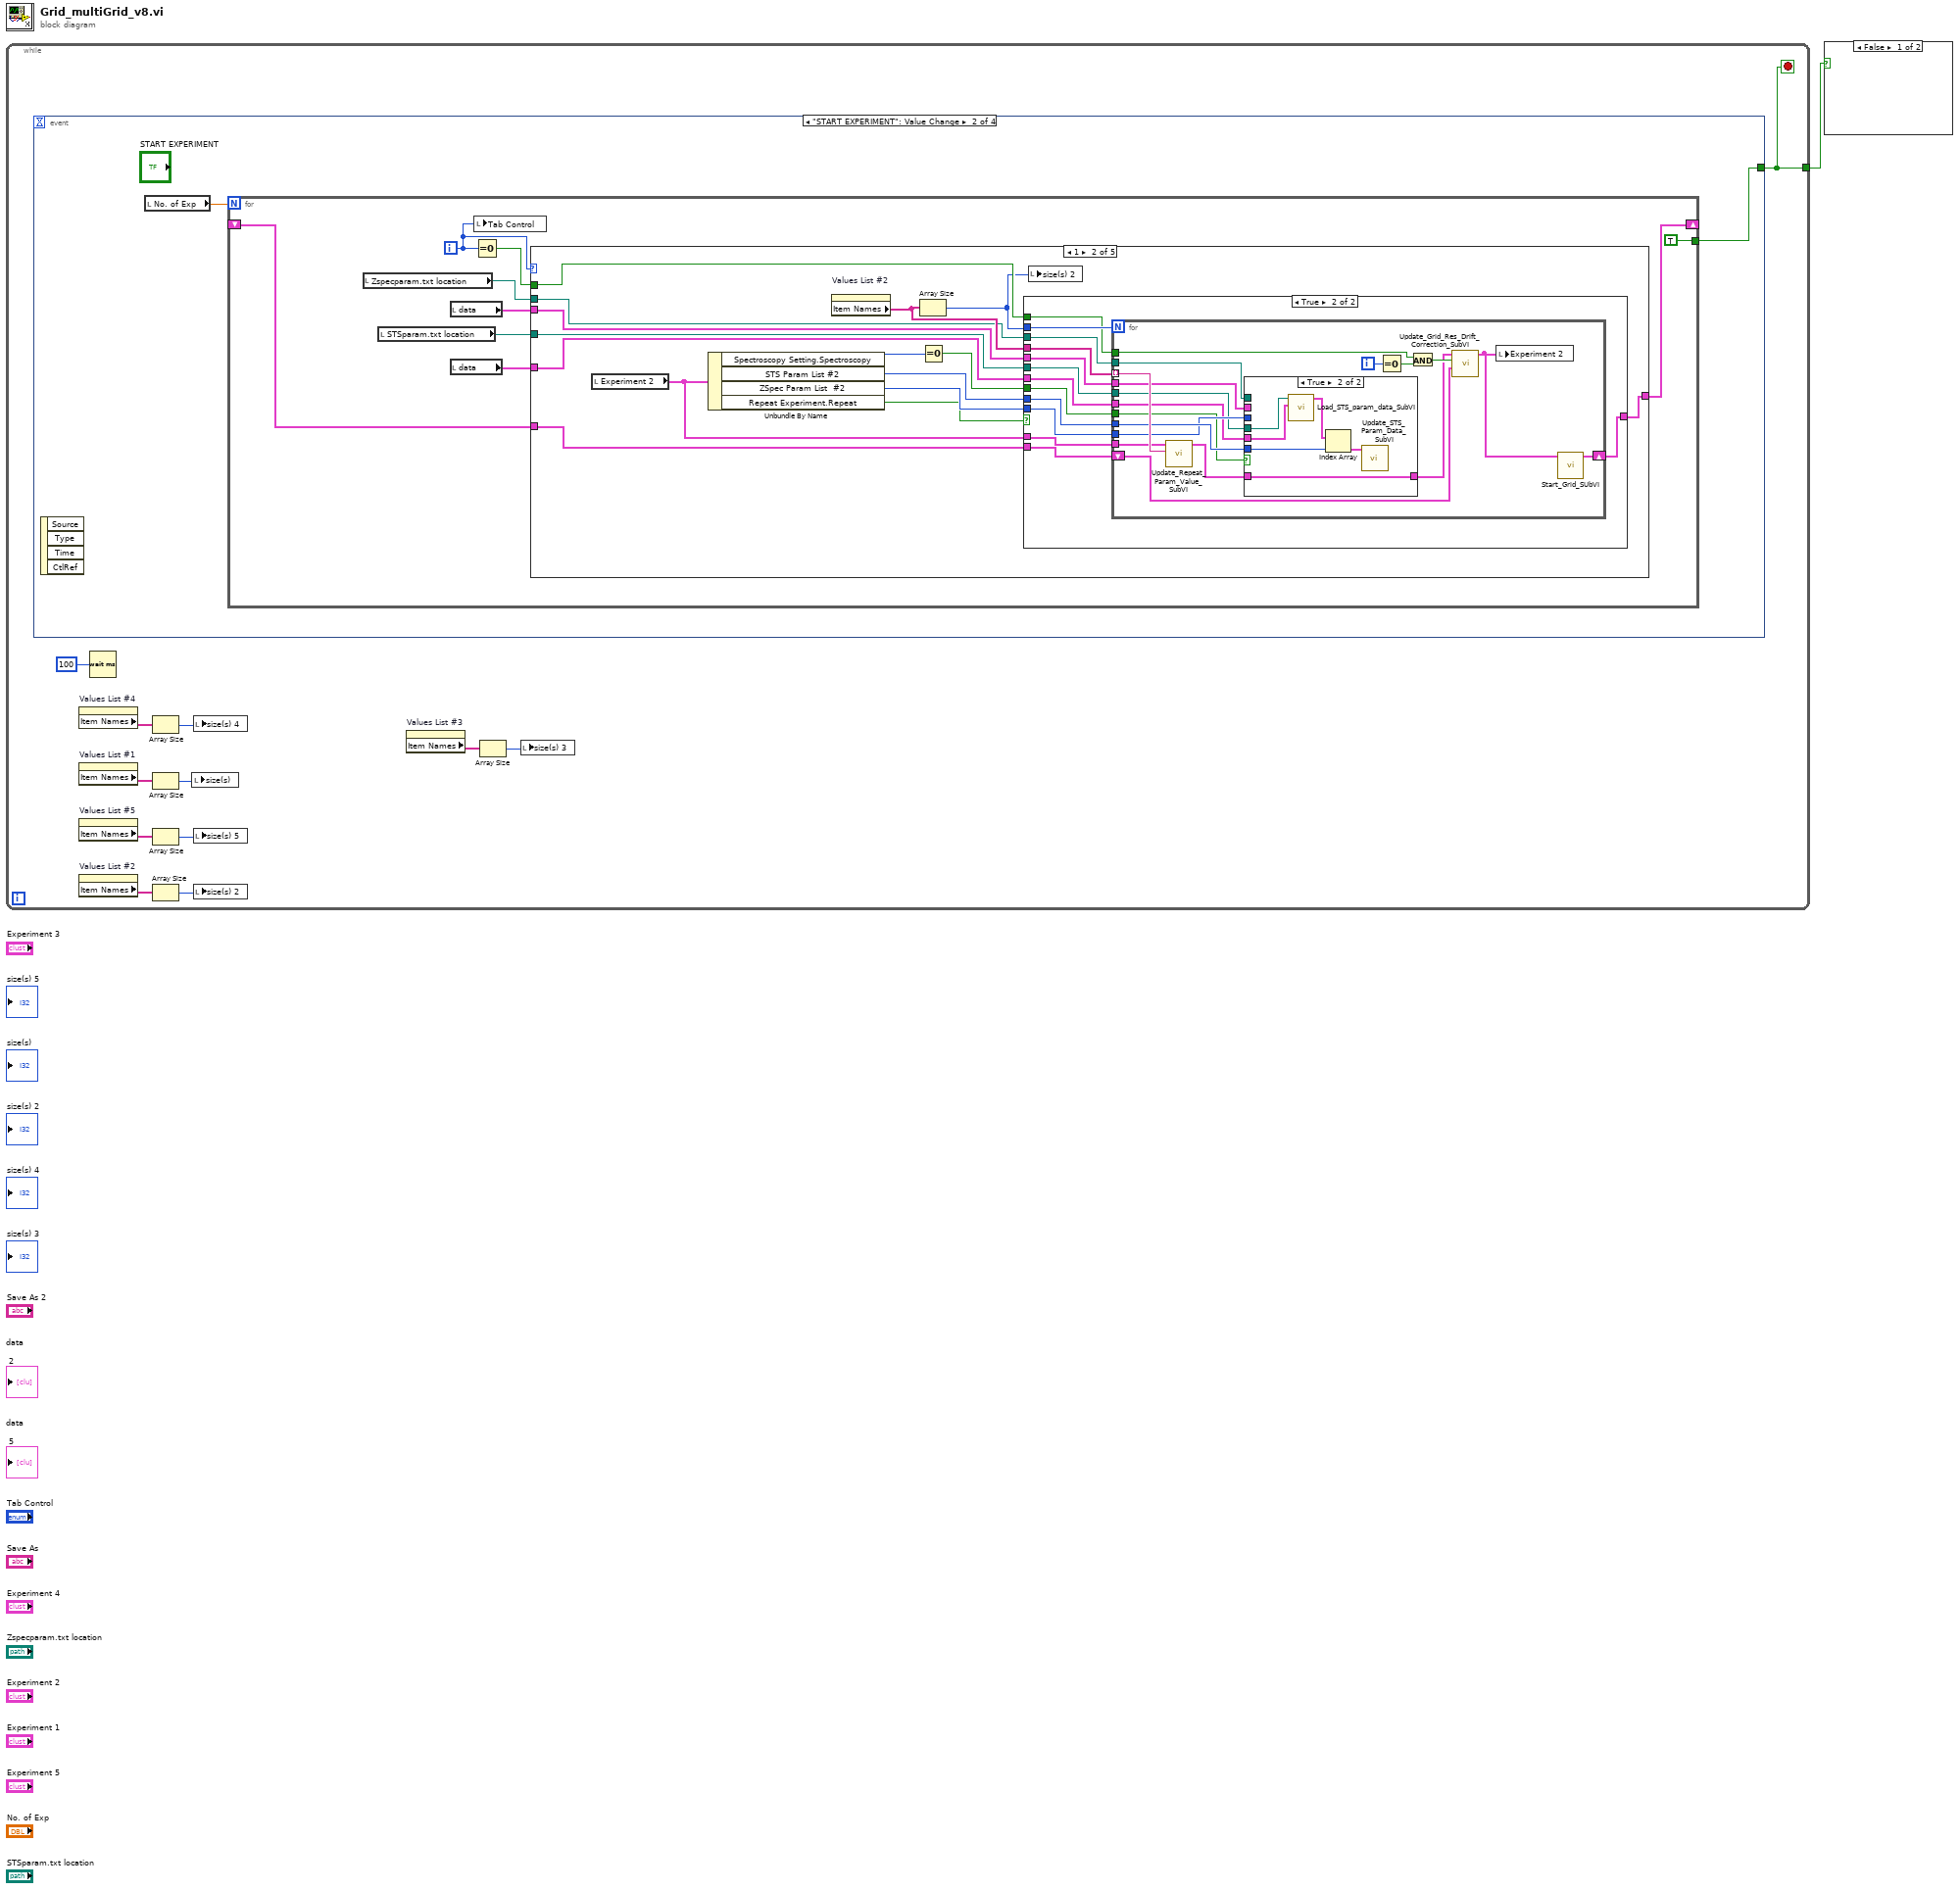
[diagram p0: block diagram]
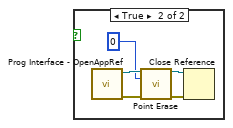
[diagram p2: hidden frame]
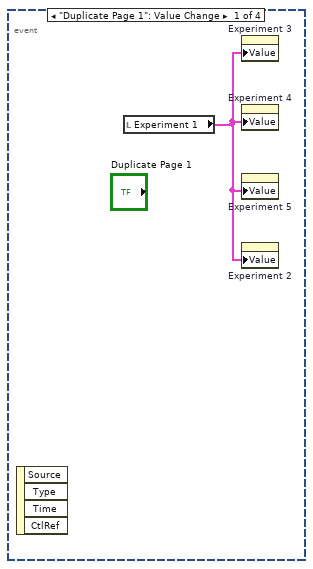
[diagram p3: hidden frame]
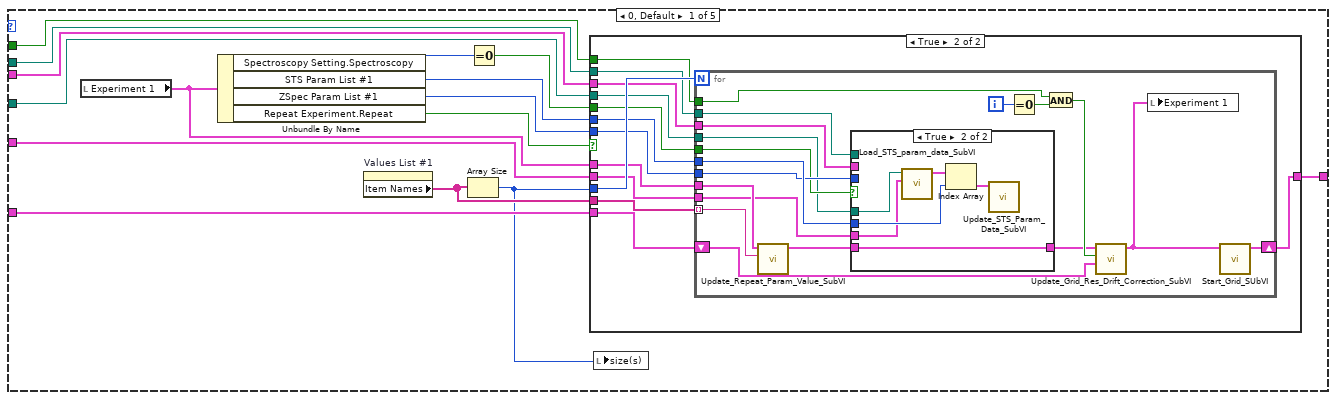
[diagram p4: hidden frame]
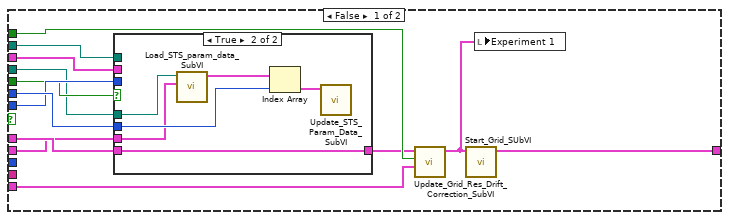
[diagram p5: hidden frame]
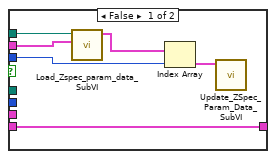
[diagram p6: hidden frame]
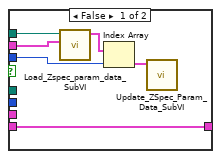
[diagram p7: hidden frame]
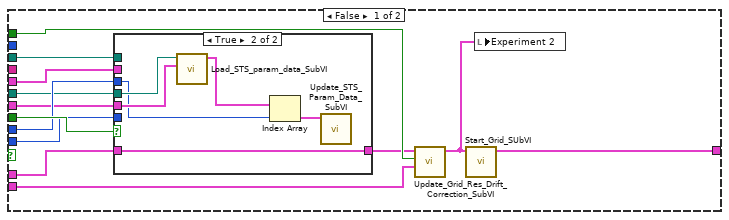
[diagram p8: hidden frame]
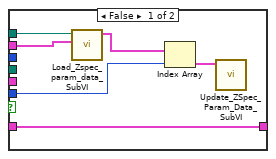
[diagram p9: hidden frame]
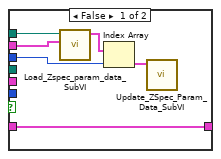
[diagram p10: hidden frame]
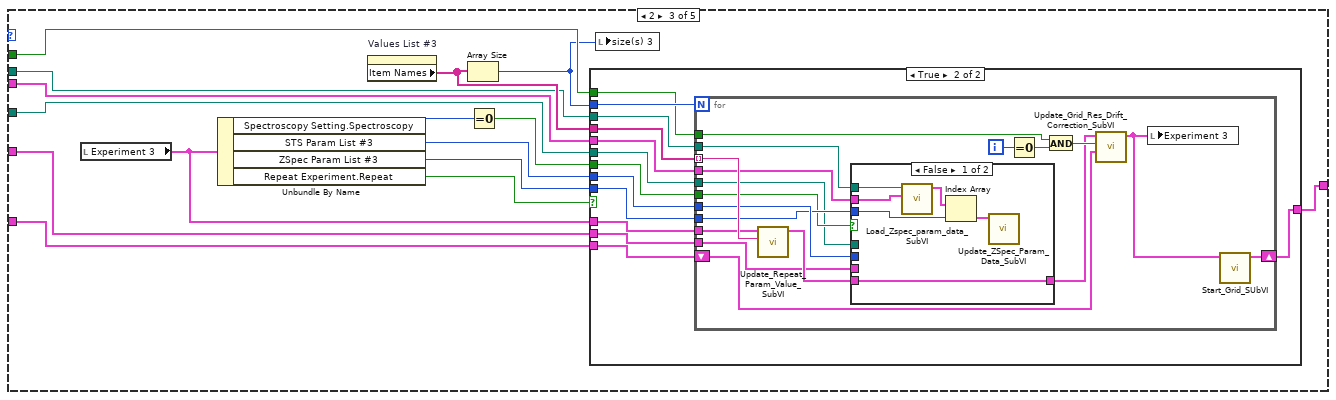
[diagram p11: hidden frame]
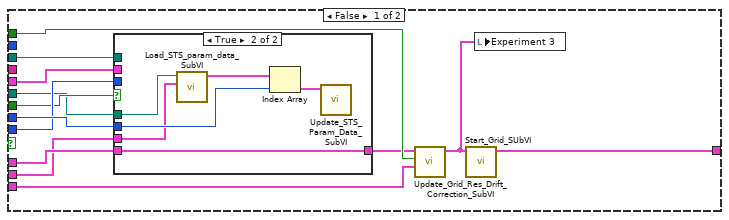
[diagram p12: hidden frame]
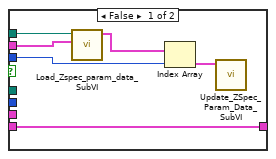
[diagram p13: hidden frame]
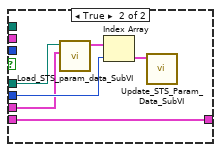
[diagram p14: hidden frame]
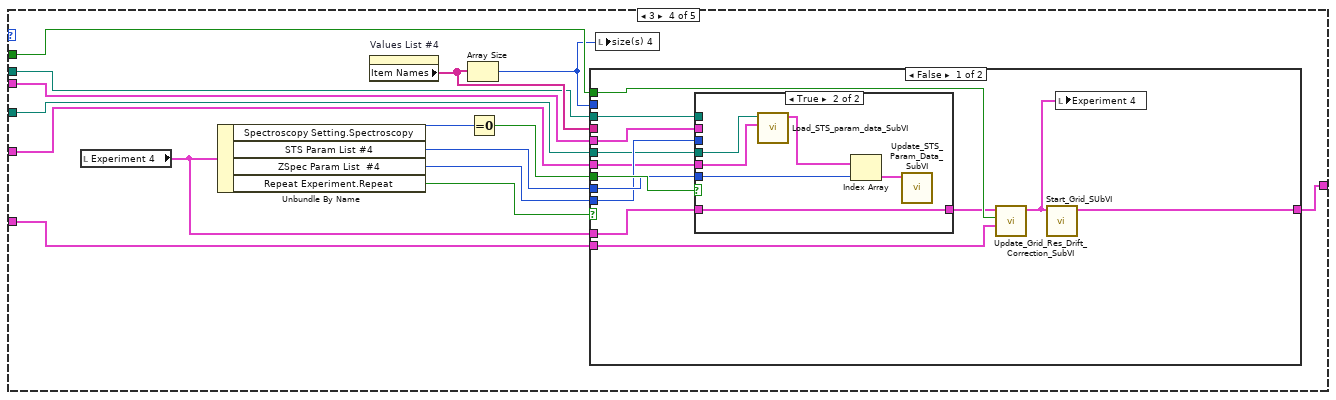
[diagram p15: hidden frame]
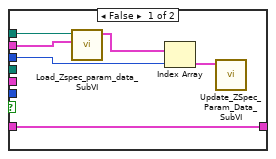
[diagram p16: hidden frame]
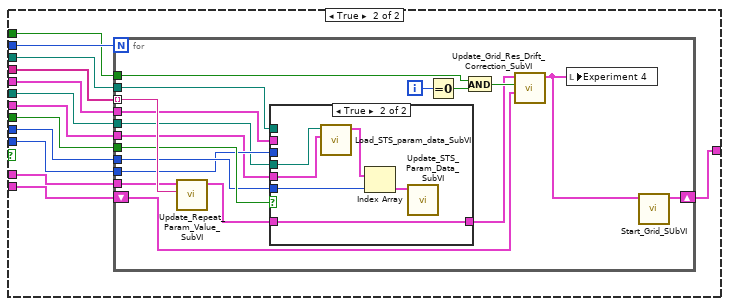
[diagram p17: hidden frame]
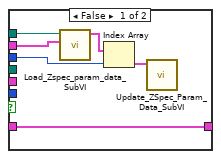
[diagram p18: hidden frame]
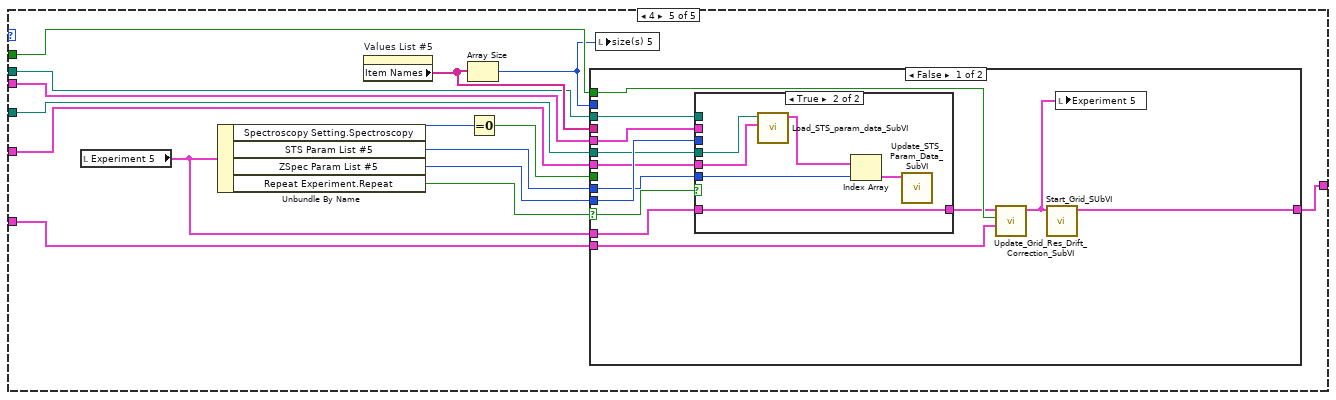
[diagram p19: hidden frame]
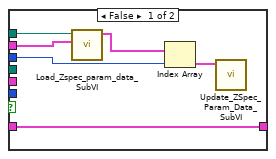
[diagram p20: hidden frame]
diagram:
  n1 = while {
    tunnel: [w12] -> w1
    stop <- w12 stop-if-true
    n2 = event shown="[1] \"START EXPERIMENT\": Value Change" {
      selector: _ -> [_ _ _ _]
      dyn-events: _ -> [_ _ _ _]
      timeout: _ -> [_ _ _ _]
      tunnel: [_ w16 _ "stop"] -> w12
      event "Duplicate Page 1": Value Change {
        n3 = event-data() -> ()  [unwired: 1 in, 4 out]
        n4 = local read "Experiment 1"() -> (w14:T4)
        n5 = property on="Experiment 3" class="Clust (strict)"("Value"=w14) -> ()  [unwired: 2 in, 2 out]
        n6 = property on="Experiment 4" class="Clust (strict)"("Value"=w14) -> ()  [unwired: 2 in, 2 out]
        n7 = property on="Experiment 5" class="Clust (strict)"("Value"=w14) -> ()  [unwired: 2 in, 2 out]
        n8 = property on="Experiment 2" class="Clust (strict)"("Value"=w14) -> ()  [unwired: 2 in, 2 out]
      }
      event "START EXPERIMENT": Value Change {
        n9 = event-data() -> ()  [unwired: 1 in, 4 out]
        n10 = local read "No. of Exp"() -> (w15:dbl)
        n11 = for {
          N: w15 -> [_]
          shift-right: [w22] -> _
          shift-left: _ -> [w24]
          tunnel: [TRUE] -> w16
          i -> [w17]
          n12 = local read "Zspecparam.txt location"() -> (w21:path)
          n13 = local read "STSparam.txt location"() -> (w20:path)
          n14 = local read "data\n\n 5"() -> (w18:T1)
          n15 = local read "data\n\n 2"() -> (w19:T2)
          n16 = local write "Tab Control"(w17) -> ()
          n17 = Equal To 0?(x=w17) -> (x = 0?=w23:bool)
          n18 = case shown="1" w17 {
            tunnel: [w40 w123 w199 w289 w372] -> w22
            tunnel: w24 -> [w34 w117 w202 w286 w371]
            tunnel: w23 -> [w33 w116 w203 w287 w370]
            tunnel: w21 -> [w29 w110 w193 w279 w361]
            tunnel: w20 -> [w30 w111 w194 w278 w362]
            tunnel: w19 -> [w28 w112 w195 w277 w360]
            tunnel: w18 -> [w27 w113 w196 w276 w359]
            frame 0, Default {
              n19 = local read "Experiment 1"() -> (w37:T4)
              n20 = Unbundle By Name(w37) -> ("Spectroscopy Setting.Spectroscopy"=w38:u16, "STS Param List #1"=w36:u16, "ZSpec Param List #1"=w35:u16, "Repeat Experiment.Repeat"=w31:bool)
              n21 = property on="Values List #1" class="LstBox (strict)"() -> ("Item Names"=w32:string[])  [unwired: 2 in, 2 out]
              n22 = Array Size(array=w32) -> (size(s)=w26:i32)
              n23 = Equal To 0?(x=w38) -> (x = 0?=w39:bool)
              n24 = case shown="True" w31 {
                tunnel: w26 -> [_ w78]
                tunnel: w37 -> [w49 w77]
                tunnel: w39 -> [w46 w76]
                tunnel: w36 -> [w50 w75]
                tunnel: w35 -> [w47 w74]
                tunnel: [w53 w73] -> w40
                tunnel: w34 -> [w52 w72]
                tunnel: w33 -> [w51 w71]
                tunnel: w32 -> [_ w70]
                tunnel: w30 -> [w43 w69]
                tunnel: w29 -> [w44 w68]
                tunnel: w28 -> [w42 w67]
                tunnel: w27 -> [w45 w66]
                frame False {
                  n25 = case shown="True" w46 {
                    tunnel: w50 -> [_ w64]
                    tunnel: w42 -> [_ w63]
                    tunnel: w43 -> [_ w62]
                    tunnel: w49 -> [w56 w60]
                    tunnel: [w56 w60] -> w48
                    tunnel: w45 -> [w58 _]
                    tunnel: w44 -> [w57 _]
                    tunnel: w47 -> [w54 _]
                    frame False {
                      n26 = call "Load_Zspec_param_data_SubVI.vi"("data\n\n 5"=w58, "Zspecparam.txt location"=w57) -> ("data"=w55:T1)  [unwired: 9 in]
                      n27 = Index Array(array=w55, index=w54) -> (element=w59:T9)
                      n28 = call "Update_ZSpec_Param_Data_SubVI.vi"("output cluster"=w59) -> ()  [unwired: 11 in]
                    }
                    frame True {
                      n29 = call "Load_STS_param_data_SubVI.vi"("data\n\n in"=w63, "STSparam.txt location"=w62) -> ("data\n\n out"=w61:T2)  [unwired: 9 in]
                      n30 = Index Array(array=w61, index=w64) -> (element=w65:T10)
                      n31 = call "Update_STS_Param_Data_SubVI.vi"("STSparameters"=w65) -> ()  [unwired: 11 in]
                    }
                  }
                  n32 = call "Update_Grid_Res_Drift_Correction_SubVI.vi"("Drift Correction Settings"=w52, "Boolean"=w51, "Experiment 6"=w48) -> ("Experiment 5"=w41:T8)  [unwired: 8 in]
                  n33 = call "Start_Grid_SUbVI.vi"("Experiment 5"=w41) -> ("Drift Correction Settings"=w53:T11)  [unwired: 10 in]
                  n34 = local write "Experiment 1"(w41) -> ()
                }
                frame True {
                  n35 = for {
                    N: w78 -> [_]
                    tunnel: w70 -> [w96] mode=indexing
                    tunnel: w77 -> [w95]
                    tunnel: w76 -> [w84]
                    tunnel: w75 -> [w86]
                    tunnel: w74 -> [w85]
                    shift-right: [w90] -> w73
                    shift-left: w72 -> [w94]
                    tunnel: w71 -> [w89]
                    tunnel: w69 -> [w83]
                    tunnel: w68 -> [w82]
                    tunnel: w67 -> [w81]
                    tunnel: w66 -> [w80]
                    i -> [w93]
                    n36 = call "Update_Repeat_Param_Value_SubVI.vi"("String"=w96, "Experiment 6"=w95) -> ("Experiment 5"=w87:T8)  [unwired: 9 in]
                    n37 = case shown="True" w84 {
                      tunnel: w86 -> [_ w107]
                      tunnel: w81 -> [_ w106]
                      tunnel: w83 -> [_ w105]
                      tunnel: w87 -> [w99 w104]
                      tunnel: [w99 w104] -> w88
                      tunnel: w80 -> [w101 _]
                      tunnel: w82 -> [w100 _]
                      tunnel: w85 -> [w97 _]
                      frame False {
                        n38 = call "Load_Zspec_param_data_SubVI.vi"("data\n\n 5"=w101, "Zspecparam.txt location"=w100) -> ("data"=w98:T1)  [unwired: 9 in]
                        n39 = Index Array(array=w98, index=w97) -> (element=w102:T9)
                        n40 = call "Update_ZSpec_Param_Data_SubVI.vi"("output cluster"=w102) -> ()  [unwired: 11 in]
                      }
                      frame True {
                        n41 = call "Load_STS_param_data_SubVI.vi"("data\n\n in"=w106, "STSparam.txt location"=w105) -> ("data\n\n out"=w103:T2)  [unwired: 9 in]
                        n42 = Index Array(array=w103, index=w107) -> (element=w108:T10)
                        n43 = call "Update_STS_Param_Data_SubVI.vi"("STSparameters"=w108) -> ()  [unwired: 11 in]
                      }
                    }
                    n44 = Equal To 0?(x=w93) -> (x = 0?=w92:bool)
                    n45 = And(x=w89, y=w92) -> (x .and. y?=w91:bool)
                    n46 = call "Update_Grid_Res_Drift_Correction_SubVI.vi"("Drift Correction Settings"=w94, "Boolean"=w91, "Experiment 6"=w88) -> ("Experiment 5"=w79:T8)  [unwired: 8 in]
                    n47 = local write "Experiment 1"(w79) -> ()
                    n48 = call "Start_Grid_SUbVI.vi"("Experiment 5"=w79) -> ("Drift Correction Settings"=w90:T11)  [unwired: 10 in]
                  }
                }
              }
              n49 = local write "size(s)"(w26) -> ()
            }
            frame 1 {
              n50 = local read "Experiment 2"() -> (w115:T5)
              n51 = Unbundle By Name(w115) -> ("Spectroscopy Setting.Spectroscopy"=w122:u16, "STS Param List #2"=w120:u16, "ZSpec Param List  #2"=w119:u16, "Repeat Experiment.Repeat"=w118:bool)
              n52 = property on="Values List #2" class="LstBox (strict)"() -> ("Item Names"=w114:string[])  [unwired: 2 in, 2 out]
              n53 = Array Size(array=w114) -> (size(s)=w109:i32)
              n54 = Equal To 0?(x=w122) -> (x = 0?=w121:bool)
              n55 = case shown="True" w118 {
                tunnel: w109 -> [_ w161]
                tunnel: w115 -> [w131 w160]
                tunnel: w121 -> [w133 w159]
                tunnel: w120 -> [w132 w158]
                tunnel: w119 -> [w129 w157]
                tunnel: [w136 w156] -> w123
                tunnel: w117 -> [w135 w155]
                tunnel: w116 -> [w134 w154]
                tunnel: w114 -> [_ w153]
                tunnel: w113 -> [w125 w152]
                tunnel: w112 -> [w126 w151]
                tunnel: w111 -> [w128 w150]
                tunnel: w110 -> [w127 w149]
                frame False {
                  n56 = case shown="True" w133 {
                    tunnel: w132 -> [_ w143]
                    tunnel: w126 -> [_ w147]
                    tunnel: w128 -> [_ w146]
                    tunnel: w131 -> [w139 w144]
                    tunnel: [w139 w144] -> w130
                    tunnel: w125 -> [w141 _]
                    tunnel: w127 -> [w140 _]
                    tunnel: w129 -> [w137 _]
                    frame False {
                      n57 = call "Load_Zspec_param_data_SubVI.vi"("data\n\n 5"=w141, "Zspecparam.txt location"=w140) -> ("data"=w138:T1)  [unwired: 9 in]
                      n58 = Index Array(array=w138, index=w137) -> (element=w142:T9)
                      n59 = call "Update_ZSpec_Param_Data_SubVI.vi"("output cluster"=w142) -> ()  [unwired: 11 in]
                    }
                    frame True {
                      n60 = call "Load_STS_param_data_SubVI.vi"("data\n\n in"=w147, "STSparam.txt location"=w146) -> ("data\n\n out"=w145:T2)  [unwired: 9 in]
                      n61 = Index Array(array=w145, index=w143) -> (element=w148:T10)
                      n62 = call "Update_STS_Param_Data_SubVI.vi"("STSparameters"=w148) -> ()  [unwired: 11 in]
                    }
                  }
                  n63 = call "Update_Grid_Res_Drift_Correction_SubVI.vi"("Drift Correction Settings"=w135, "Boolean"=w134, "Experiment 6"=w130) -> ("Experiment 5"=w124:T8)  [unwired: 8 in]
                  n64 = call "Start_Grid_SUbVI.vi"("Experiment 5"=w124) -> ("Drift Correction Settings"=w136:T11)  [unwired: 10 in]
                  n65 = local write "Experiment 2"(w124) -> ()
                }
                frame True {
                  n66 = for {
                    N: w161 -> [_]
                    tunnel: w153 -> [w179] mode=indexing
                    tunnel: w160 -> [w178]
                    tunnel: w159 -> [w169]
                    tunnel: w158 -> [w171]
                    tunnel: w157 -> [w170]
                    shift-right: [w173] -> w156
                    shift-left: w155 -> [w177]
                    tunnel: w154 -> [w172]
                    tunnel: w152 -> [w166]
                    tunnel: w151 -> [w165]
                    tunnel: w150 -> [w164]
                    tunnel: w149 -> [w163]
                    i -> [w176]
                    n67 = call "Update_Repeat_Param_Value_SubVI.vi"("String"=w179, "Experiment 6"=w178) -> ("Experiment 5"=w168:T8)  [unwired: 9 in]
                    n68 = case shown="True" w169 {
                      tunnel: w171 -> [_ w190]
                      tunnel: w165 -> [_ w189]
                      tunnel: w164 -> [_ w188]
                      tunnel: w168 -> [w182 w187]
                      tunnel: [w182 w187] -> w167
                      tunnel: w166 -> [w184 _]
                      tunnel: w163 -> [w183 _]
                      tunnel: w170 -> [w180 _]
                      frame False {
                        n69 = call "Load_Zspec_param_data_SubVI.vi"("data\n\n 5"=w184, "Zspecparam.txt location"=w183) -> ("data"=w181:T1)  [unwired: 9 in]
                        n70 = Index Array(array=w181, index=w180) -> (element=w185:T9)
                        n71 = call "Update_ZSpec_Param_Data_SubVI.vi"("output cluster"=w185) -> ()  [unwired: 11 in]
                      }
                      frame True {
                        n72 = call "Load_STS_param_data_SubVI.vi"("data\n\n in"=w189, "STSparam.txt location"=w188) -> ("data\n\n out"=w186:T2)  [unwired: 9 in]
                        n73 = Index Array(array=w186, index=w190) -> (element=w191:T10)
                        n74 = call "Update_STS_Param_Data_SubVI.vi"("STSparameters"=w191) -> ()  [unwired: 11 in]
                      }
                    }
                    n75 = Equal To 0?(x=w176) -> (x = 0?=w175:bool)
                    n76 = And(x=w172, y=w175) -> (x .and. y?=w174:bool)
                    n77 = call "Update_Grid_Res_Drift_Correction_SubVI.vi"("Drift Correction Settings"=w177, "Boolean"=w174, "Experiment 6"=w167) -> ("Experiment 5"=w162:T8)  [unwired: 8 in]
                    n78 = local write "Experiment 2"(w162) -> ()
                    n79 = call "Start_Grid_SUbVI.vi"("Experiment 5"=w162) -> ("Drift Correction Settings"=w173:T11)  [unwired: 10 in]
                  }
                }
              }
              n80 = local write "size(s) 2"(w109) -> ()
            }
            frame 2 {
              n81 = local read "Experiment 3"() -> (w200:T6)
              n82 = Unbundle By Name(w200) -> ("Spectroscopy Setting.Spectroscopy"=w197:u16, "STS Param List #3"=w206:u16, "ZSpec Param List #3"=w205:u16, "Repeat Experiment.Repeat"=w204:bool)
              n83 = property on="Values List #3" class="LstBox (strict)"() -> ("Item Names"=w201:string[])  [unwired: 2 in, 2 out]
              n84 = Array Size(array=w201) -> (size(s)=w192:i32)
              n85 = Equal To 0?(x=w197) -> (x = 0?=w198:bool)
              n86 = case shown="True" w204 {
                tunnel: w192 -> [_ w244]
                tunnel: w200 -> [w215 w243]
                tunnel: w198 -> [w212 w242]
                tunnel: w206 -> [w214 w241]
                tunnel: w205 -> [w213 w240]
                tunnel: [w217 w239] -> w199
                tunnel: w202 -> [w219 w238]
                tunnel: w203 -> [w218 w237]
                tunnel: w201 -> [_ w236]
                tunnel: w196 -> [w211 w232]
                tunnel: w195 -> [w210 w235]
                tunnel: w194 -> [w209 w233]
                tunnel: w193 -> [w208 w234]
                frame False {
                  n87 = case shown="True" w212 {
                    tunnel: w214 -> [_ w230]
                    tunnel: w210 -> [_ w229]
                    tunnel: w209 -> [_ w228]
                    tunnel: w215 -> [w222 w227]
                    tunnel: [w222 w227] -> w216
                    tunnel: w211 -> [w224 _]
                    tunnel: w208 -> [w223 _]
                    tunnel: w213 -> [w220 _]
                    frame False {
                      n88 = call "Load_Zspec_param_data_SubVI.vi"("data\n\n 5"=w224, "Zspecparam.txt location"=w223) -> ("data"=w221:T1)  [unwired: 9 in]
                      n89 = Index Array(array=w221, index=w220) -> (element=w225:T9)
                      n90 = call "Update_ZSpec_Param_Data_SubVI.vi"("output cluster"=w225) -> ()  [unwired: 11 in]
                    }
                    frame True {
                      n91 = call "Load_STS_param_data_SubVI.vi"("data\n\n in"=w229, "STSparam.txt location"=w228) -> ("data\n\n out"=w226:T2)  [unwired: 9 in]
                      n92 = Index Array(array=w226, index=w230) -> (element=w231:T10)
                      n93 = call "Update_STS_Param_Data_SubVI.vi"("STSparameters"=w231) -> ()  [unwired: 11 in]
                    }
                  }
                  n94 = call "Update_Grid_Res_Drift_Correction_SubVI.vi"("Drift Correction Settings"=w219, "Boolean"=w218, "Experiment 6"=w216) -> ("Experiment 5"=w207:T8)  [unwired: 8 in]
                  n95 = call "Start_Grid_SUbVI.vi"("Experiment 5"=w207) -> ("Drift Correction Settings"=w217:T11)  [unwired: 10 in]
                  n96 = local write "Experiment 3"(w207) -> ()
                }
                frame True {
                  n97 = for {
                    N: w244 -> [_]
                    tunnel: w236 -> [w262] mode=indexing
                    tunnel: w243 -> [w261]
                    tunnel: w242 -> [w250]
                    tunnel: w241 -> [w252]
                    tunnel: w240 -> [w251]
                    shift-right: [w256] -> w239
                    shift-left: w238 -> [w260]
                    tunnel: w237 -> [w255]
                    tunnel: w235 -> [w249]
                    tunnel: w234 -> [w248]
                    tunnel: w233 -> [w247]
                    tunnel: w232 -> [w246]
                    i -> [w259]
                    n98 = call "Update_Repeat_Param_Value_SubVI.vi"("String"=w262, "Experiment 6"=w261) -> ("Experiment 5"=w254:T8)  [unwired: 9 in]
                    n99 = case shown="False" w250 {
                      tunnel: w252 -> [_ w273]
                      tunnel: w249 -> [_ w272]
                      tunnel: w247 -> [_ w271]
                      tunnel: w254 -> [w265 w270]
                      tunnel: [w265 w270] -> w253
                      tunnel: w246 -> [w267 _]
                      tunnel: w248 -> [w266 _]
                      tunnel: w251 -> [w263 _]
                      frame False {
                        n100 = call "Load_Zspec_param_data_SubVI.vi"("data\n\n 5"=w267, "Zspecparam.txt location"=w266) -> ("data"=w264:T1)  [unwired: 9 in]
                        n101 = Index Array(array=w264, index=w263) -> (element=w268:T9)
                        n102 = call "Update_ZSpec_Param_Data_SubVI.vi"("output cluster"=w268) -> ()  [unwired: 11 in]
                      }
                      frame True {
                        n103 = call "Load_STS_param_data_SubVI.vi"("data\n\n in"=w272, "STSparam.txt location"=w271) -> ("data\n\n out"=w269:T2)  [unwired: 9 in]
                        n104 = Index Array(array=w269, index=w273) -> (element=w274:T10)
                        n105 = call "Update_STS_Param_Data_SubVI.vi"("STSparameters"=w274) -> ()  [unwired: 11 in]
                      }
                    }
                    n106 = Equal To 0?(x=w259) -> (x = 0?=w258:bool)
                    n107 = And(x=w255, y=w258) -> (x .and. y?=w257:bool)
                    n108 = call "Update_Grid_Res_Drift_Correction_SubVI.vi"("Drift Correction Settings"=w260, "Boolean"=w257, "Experiment 6"=w253) -> ("Experiment 5"=w245:T8)  [unwired: 8 in]
                    n109 = local write "Experiment 3"(w245) -> ()
                    n110 = call "Start_Grid_SUbVI.vi"("Experiment 5"=w245) -> ("Drift Correction Settings"=w256:T11)  [unwired: 10 in]
                  }
                }
              }
              n111 = local write "size(s) 3"(w192) -> ()
            }
            frame 3 {
              n112 = local read "Experiment 4"() -> (w284:T7)
              n113 = Unbundle By Name(w284) -> ("Spectroscopy Setting.Spectroscopy"=w281:u16, "STS Param List #4"=w282:u16, "ZSpec Param List  #4"=w283:u16, "Repeat Experiment.Repeat"=w288:bool)
              n114 = property on="Values List #4" class="LstBox (strict)"() -> ("Item Names"=w285:string[])  [unwired: 2 in, 2 out]
              n115 = Array Size(array=w285) -> (size(s)=w275:i32)
              n116 = Equal To 0?(x=w281) -> (x = 0?=w280:bool)
              n117 = case shown="False" w288 {
                tunnel: w275 -> [_ w327]
                tunnel: w284 -> [w298 w326]
                tunnel: w280 -> [w297 w325]
                tunnel: w282 -> [w296 w324]
                tunnel: w283 -> [w295 w323]
                tunnel: [w302 w322] -> w289
                tunnel: w286 -> [w301 w321]
                tunnel: w287 -> [w300 w320]
                tunnel: w285 -> [_ w319]
                tunnel: w279 -> [w293 w318]
                tunnel: w278 -> [w294 w317]
                tunnel: w277 -> [w292 w316]
                tunnel: w276 -> [w291 w315]
                frame False {
                  n118 = case shown="True" w297 {
                    tunnel: w296 -> [_ w313]
                    tunnel: w292 -> [_ w312]
                    tunnel: w294 -> [_ w311]
                    tunnel: w298 -> [w305 w310]
                    tunnel: [w305 w310] -> w299
                    tunnel: w291 -> [w307 _]
                    tunnel: w293 -> [w306 _]
                    tunnel: w295 -> [w303 _]
                    frame False {
                      n119 = call "Load_Zspec_param_data_SubVI.vi"("data\n\n 5"=w307, "Zspecparam.txt location"=w306) -> ("data"=w304:T1)  [unwired: 9 in]
                      n120 = Index Array(array=w304, index=w303) -> (element=w308:T9)
                      n121 = call "Update_ZSpec_Param_Data_SubVI.vi"("output cluster"=w308) -> ()  [unwired: 11 in]
                    }
                    frame True {
                      n122 = call "Load_STS_param_data_SubVI.vi"("data\n\n in"=w312, "STSparam.txt location"=w311) -> ("data\n\n out"=w309:T2)  [unwired: 9 in]
                      n123 = Index Array(array=w309, index=w313) -> (element=w314:T10)
                      n124 = call "Update_STS_Param_Data_SubVI.vi"("STSparameters"=w314) -> ()  [unwired: 11 in]
                    }
                  }
                  n125 = call "Update_Grid_Res_Drift_Correction_SubVI.vi"("Drift Correction Settings"=w301, "Boolean"=w300, "Experiment 6"=w299) -> ("Experiment 5"=w290:T8)  [unwired: 8 in]
                  n126 = call "Start_Grid_SUbVI.vi"("Experiment 5"=w290) -> ("Drift Correction Settings"=w302:T11)  [unwired: 10 in]
                  n127 = local write "Experiment 4"(w290) -> ()
                }
                frame True {
                  n128 = for {
                    N: w327 -> [_]
                    tunnel: w319 -> [w345] mode=indexing
                    tunnel: w326 -> [w344]
                    tunnel: w325 -> [w335]
                    tunnel: w324 -> [w334]
                    tunnel: w323 -> [w333]
                    shift-right: [w339] -> w322
                    shift-left: w321 -> [w343]
                    tunnel: w320 -> [w338]
                    tunnel: w318 -> [w332]
                    tunnel: w317 -> [w331]
                    tunnel: w316 -> [w330]
                    tunnel: w315 -> [w329]
                    i -> [w342]
                    n129 = call "Update_Repeat_Param_Value_SubVI.vi"("String"=w345, "Experiment 6"=w344) -> ("Experiment 5"=w337:T8)  [unwired: 9 in]
                    n130 = case shown="True" w335 {
                      tunnel: w334 -> [_ w356]
                      tunnel: w330 -> [_ w355]
                      tunnel: w331 -> [_ w354]
                      tunnel: w337 -> [w346 w352]
                      tunnel: w329 -> [w350 _]
                      tunnel: w332 -> [w349 _]
                      tunnel: w333 -> [w347 _]
                      tunnel: [w346 w352] -> w336
                      frame False {
                        n131 = call "Load_Zspec_param_data_SubVI.vi"("data\n\n 5"=w350, "Zspecparam.txt location"=w349) -> ("data"=w348:T1)  [unwired: 9 in]
                        n132 = Index Array(array=w348, index=w347) -> (element=w351:T9)
                        n133 = call "Update_ZSpec_Param_Data_SubVI.vi"("output cluster"=w351) -> ()  [unwired: 11 in]
                      }
                      frame True {
                        n134 = call "Load_STS_param_data_SubVI.vi"("data\n\n in"=w355, "STSparam.txt location"=w354) -> ("data\n\n out"=w353:T2)  [unwired: 9 in]
                        n135 = Index Array(array=w353, index=w356) -> (element=w357:T10)
                        n136 = call "Update_STS_Param_Data_SubVI.vi"("STSparameters"=w357) -> ()  [unwired: 11 in]
                      }
                    }
                    n137 = Equal To 0?(x=w342) -> (x = 0?=w341:bool)
                    n138 = And(x=w338, y=w341) -> (x .and. y?=w340:bool)
                    n139 = call "Update_Grid_Res_Drift_Correction_SubVI.vi"("Drift Correction Settings"=w343, "Boolean"=w340, "Experiment 6"=w336) -> ("Experiment 5"=w328:T8)  [unwired: 8 in]
                    n140 = local write "Experiment 4"(w328) -> ()
                    n141 = call "Start_Grid_SUbVI.vi"("Experiment 5"=w328) -> ("Drift Correction Settings"=w339:T11)  [unwired: 10 in]
                  }
                }
              }
              n142 = local write "size(s) 4"(w275) -> ()
            }
            frame 4 {
              n143 = local read "Experiment 5"() -> (w367:T8)
              n144 = Unbundle By Name(w367) -> ("Spectroscopy Setting.Spectroscopy"=w363:u16, "STS Param List #5"=w365:u16, "ZSpec Param List #5"=w366:u16, "Repeat Experiment.Repeat"=w369:bool)
              n145 = property on="Values List #5" class="LstBox (strict)"() -> ("Item Names"=w368:string[])  [unwired: 2 in, 2 out]
              n146 = Array Size(array=w368) -> (size(s)=w358:i32)
              n147 = Equal To 0?(x=w363) -> (x = 0?=w364:bool)
              n148 = case shown="False" w369 {
                selector: w369 -> [w380 _]
                tunnel: w358 -> [_ w410]
                tunnel: w367 -> [w378 w409]
                tunnel: w364 -> [_ w408]
                tunnel: w365 -> [w381 w407]
                tunnel: w366 -> [w382 w406]
                tunnel: [w385 w405] -> w372
                tunnel: w371 -> [w384 w404]
                tunnel: w370 -> [w383 w403]
                tunnel: w368 -> [_ w402]
                tunnel: w362 -> [w377 w401]
                tunnel: w361 -> [w376 w400]
                tunnel: w360 -> [w375 w399]
                tunnel: w359 -> [w374 w398]
                frame False {
                  n149 = case shown="True" w380 {
                    tunnel: w381 -> [_ w396]
                    tunnel: w375 -> [_ w395]
                    tunnel: w377 -> [_ w394]
                    tunnel: w378 -> [w388 w392]
                    tunnel: [w388 w392] -> w379
                    tunnel: w374 -> [w390 _]
                    tunnel: w376 -> [w389 _]
                    tunnel: w382 -> [w386 _]
                    frame False {
                      n150 = call "Load_Zspec_param_data_SubVI.vi"("data\n\n 5"=w390, "Zspecparam.txt location"=w389) -> ("data"=w387:T1)  [unwired: 9 in]
                      n151 = Index Array(array=w387, index=w386) -> (element=w391:T9)
                      n152 = call "Update_ZSpec_Param_Data_SubVI.vi"("output cluster"=w391) -> ()  [unwired: 11 in]
                    }
                    frame True {
                      n153 = call "Load_STS_param_data_SubVI.vi"("data\n\n in"=w395, "STSparam.txt location"=w394) -> ("data\n\n out"=w393:T2)  [unwired: 9 in]
                      n154 = Index Array(array=w393, index=w396) -> (element=w397:T10)
                      n155 = call "Update_STS_Param_Data_SubVI.vi"("STSparameters"=w397) -> ()  [unwired: 11 in]
                    }
                  }
                  n156 = call "Update_Grid_Res_Drift_Correction_SubVI.vi"("Drift Correction Settings"=w384, "Boolean"=w383, "Experiment 6"=w379) -> ("Experiment 5"=w373:T8)  [unwired: 8 in]
                  n157 = call "Start_Grid_SUbVI.vi"("Experiment 5"=w373) -> ("Drift Correction Settings"=w385:T11)  [unwired: 10 in]
                  n158 = local write "Experiment 5"(w373) -> ()
                }
                frame True {
                  n159 = for {
                    N: w410 -> [_]
                    tunnel: w402 -> [w428] mode=indexing
                    tunnel: w409 -> [w427]
                    tunnel: w408 -> [w416]
                    tunnel: w407 -> [w417]
                    tunnel: w406 -> [w418]
                    shift-right: [w422] -> w405
                    shift-left: w404 -> [w426]
                    tunnel: w403 -> [w421]
                    tunnel: w401 -> [w415]
                    tunnel: w400 -> [w414]
                    tunnel: w399 -> [w413]
                    tunnel: w398 -> [w412]
                    i -> [w425]
                    n160 = call "Update_Repeat_Param_Value_SubVI.vi"("String"=w428, "Experiment 6"=w427) -> ("Experiment 5"=w420:T8)  [unwired: 9 in]
                    n161 = case shown="True" w416 {
                      tunnel: w417 -> [_ w439]
                      tunnel: w413 -> [_ w438]
                      tunnel: w415 -> [_ w437]
                      tunnel: w420 -> [w431 w436]
                      tunnel: [w431 w436] -> w419
                      tunnel: w412 -> [w433 _]
                      tunnel: w414 -> [w432 _]
                      tunnel: w418 -> [w429 _]
                      frame False {
                        n162 = call "Load_Zspec_param_data_SubVI.vi"("data\n\n 5"=w433, "Zspecparam.txt location"=w432) -> ("data"=w430:T1)  [unwired: 9 in]
                        n163 = Index Array(array=w430, index=w429) -> (element=w434:T9)
                        n164 = call "Update_ZSpec_Param_Data_SubVI.vi"("output cluster"=w434) -> ()  [unwired: 11 in]
                      }
                      frame True {
                        n165 = call "Load_STS_param_data_SubVI.vi"("data\n\n in"=w438, "STSparam.txt location"=w437) -> ("data\n\n out"=w435:T2)  [unwired: 9 in]
                        n166 = Index Array(array=w435, index=w439) -> (element=w440:T10)
                        n167 = call "Update_STS_Param_Data_SubVI.vi"("STSparameters"=w440) -> ()  [unwired: 11 in]
                      }
                    }
                    n168 = Equal To 0?(x=w425) -> (x = 0?=w424:bool)
                    n169 = And(x=w421, y=w424) -> (x .and. y?=w423:bool)
                    n170 = call "Update_Grid_Res_Drift_Correction_SubVI.vi"("Drift Correction Settings"=w426, "Boolean"=w423, "Experiment 6"=w419) -> ("Experiment 5"=w411:T8)  [unwired: 8 in]
                    n171 = local write "Experiment 5"(w411) -> ()
                    n172 = call "Start_Grid_SUbVI.vi"("Experiment 5"=w411) -> ("Drift Correction Settings"=w422:T11)  [unwired: 10 in]
                  }
                }
              }
              n173 = local write "size(s) 5"(w358) -> ()
            }
          }
        }
      }
      event "Update STS/Zspec Param List": Value Change {
        n174 = event-data() -> ()  [unwired: 1 in, 6 out]
        n175 = local read "STSparam.txt location"() -> (w447:path)
        n176 = local read "Zspecparam.txt location"() -> (w446:path)
        n177 = control-ref of="data\n\n 2"() -> (w445:refnum<vi>)
        n178 = call "Load_STS_param_options_SubVI.vi"("STSparam.txt location"=w447, "Array in"=w445) -> ("error out"=w448:errorcluster, "Array"=w442:string[])  [unwired: 8 in]
        n179 = control-ref of="data\n\n 5"() -> (w444:refnum<vi>)
        n180 = call "Load_Zspec_param_options_SubVI.vi"("error in (no error)"=w448, "Zspecparam.txt location"=w446, "Array in"=w444) -> ("Array"=w443:string[])  [unwired: 8 in]
        n181 = for {
          N: 5 -> [_]
          tunnel: w443 -> [w450]
          tunnel: w442 -> [w449]
          i -> [w451]
          n182 = case shown="0, Default" w451 {
            tunnel: w450 -> [w453 w455 w457 w459 w461]
            tunnel: w449 -> [w452 w454 w456 w458 w460]
            frame 0, Default {
              n183 = property on="STS Param List #1" class="Ring (strict)"("Strings []"=w452) -> ()  [unwired: 2 in, 2 out]
              n184 = property on="ZSpec Param List #1" class="Ring (strict)"("Strings []"=w453) -> ()  [unwired: 2 in, 2 out]
            }
            frame 1 {
              n185 = property on="STS Param List #2" class="Ring (strict)"("Strings []"=w454) -> ()  [unwired: 2 in, 2 out]
              n186 = property on="ZSpec Param List  #2" class="Ring (strict)"("Strings []"=w455) -> ()  [unwired: 2 in, 2 out]
            }
            frame 2 {
              n187 = property on="STS Param List #3" class="Ring (strict)"("Strings []"=w456) -> ()  [unwired: 2 in, 2 out]
              n188 = property on="ZSpec Param List #3" class="Ring (strict)"("Strings []"=w457) -> ()  [unwired: 2 in, 2 out]
            }
            frame 3 {
              n189 = property on="STS Param List #4" class="Ring (strict)"("Strings []"=w458) -> ()  [unwired: 2 in, 2 out]
              n190 = property on="ZSpec Param List  #4" class="Ring (strict)"("Strings []"=w459) -> ()  [unwired: 2 in, 2 out]
            }
            frame 4 {
              n191 = property on="STS Param List #5" class="Ring (strict)"("Strings []"=w460) -> ()  [unwired: 2 in, 2 out]
              n192 = property on="ZSpec Param List #5" class="Ring (strict)"("Strings []"=w461) -> ()  [unwired: 2 in, 2 out]
            }
          }
        }
      }
      event "stop": Value Change {
        n193 = event-data() -> ()  [unwired: 1 in, 4 out]
      }
    }
    n194 = property on="Values List #4" class="LstBox (strict)"() -> ("Item Names"=w3:string[])  [unwired: 2 in, 2 out]
    n195 = property on="Values List #1" class="LstBox (strict)"() -> ("Item Names"=w6:string[])  [unwired: 2 in, 2 out]
    n196 = property on="Values List #5" class="LstBox (strict)"() -> ("Item Names"=w2:string[])  [unwired: 2 in, 2 out]
    n197 = property on="Values List #2" class="LstBox (strict)"() -> ("Item Names"=w5:string[])  [unwired: 2 in, 2 out]
    n198 = Wait (ms)(milliseconds to wait=u32 100) -> ()  [unwired: 1 out]
    n199 = Array Size(array=w3) -> (size(s)=w8:i32)
    n200 = Array Size(array=w6) -> (size(s)=w11:i32)
    n201 = Array Size(array=w2) -> (size(s)=w7:i32)
    n202 = Array Size(array=w5) -> (size(s)=w10:i32)
    n203 = local write "size(s)"(w11) -> ()
    n204 = local write "size(s) 4"(w8) -> ()
    n205 = local write "size(s) 5"(w7) -> ()
    n206 = local write "size(s) 2"(w10) -> ()
    n207 = property on="Values List #3" class="LstBox (strict)"() -> ("Item Names"=w4:string[])  [unwired: 2 in, 2 out]
    n208 = Array Size(array=w4) -> (size(s)=w9:i32)
    n209 = local write "size(s) 3"(w9) -> ()
  }
  n210 = case shown="False" w1 {
    frame False {
    }
    frame True {
      n211 = call <userlib>:"Prog Interface - OpenAppRef.vi"() -> ("Error out"=w466:errorcluster, "Application reference"=w467:refnum<vi>)  [unwired: 6 in]
      n212 = call <userlib>:"Point Erase.vi"("Application ref in"=w467, "Point index (-1=All points)"=0, "error in (no error)"=w466) -> ("Application ref out"=w463:refnum<vi>, "error out"=w464:errorcluster)  [unwired: 11 in]
      n213 = Close Reference(reference=w463, error in (no error)=w464) -> ()  [unwired: 1 out]
    }
  }
